vi "Notebooks JSON to LV.vi"(8 "error in (no error)":errorcluster, 11 "Notebooks JSON":string="{\r\n  \"@odata.context\":\"https://www.onenote.com/api/v1.0/$metadata#me/notes/notebooks\",\"value\":[\r\n    {\r\n      \"id\":\"0-C3A40648AD0C9170!191210\",\"self\":\"https://www.onenote.com/api/v1.0/me/notes/notebooks/0-C3A40648AD0C9170!191210\",\"createdTime\":\"2013-11-06T13:59:29.113Z\",\"name\":\"1st Floor Touchscreen\",\"createdBy\":\"Ansom Voodoo\",\"lastModifiedBy\":\"Ansom Voodoo\",\"lastModifiedTime\":\"2018-04-10T18:41:37.72Z\",\"isDefault\":false,\"userRole\":\"Contributor\",\"isShared\":true,\"sectionsUrl\":\"https://www.onenote.com/api/v1.0/me/notes/notebooks/0-C3A40648AD0C9170!191210/sections\",\"sectionGroupsUrl\":\"https://www.onenote.com/api/v1.0/me/notes/notebooks/0-C3A40648AD0C9170!191210/sectionGroups\",\"links\":{\r\n        \"oneNoteClientUrl\":{\r\n          \"href\":\"onenote:https://d.docs.live.net/c3a40648ad0c9170/ansom/Expt.ansom/TouchScreens/1st%20Floor%20Touchscreen\"\r\n        },\"oneNoteWebUrl\":{\r\n          \"href\":\"https://onedrive.live.com/redir.aspx?cid=c3a40648ad0c9170&page=edit&resid=C3A40648AD0C9170!191210&parId=C3A40648AD0C9170!191178\"\r\n        }\r\n      }\r\n    },{\r\n      \"id\":\"0-C3A40648AD0C9170!51956\",\"self\":\"https://www.onenote.com/api/v1.0/me/notes/notebooks/0-C3A40648AD0C9170!51956\",\"createdTime\":\"2013-10-21T12:23:03.47Z\",\"name\":\"2nd Floor TouchScreen\",\"createdBy\":\"Ansom Voodoo\",\"lastModifiedBy\":\"Ansom Voodoo\",\"lastModifiedTime\":\"2018-04-09T20:16:56.763Z\",\"isDefault\":false,\"userRole\":\"Contributor\",\"isShared\":true,\"sectionsUrl\":\"https://www.onenote.com/api/v1.0/me/notes/notebooks/0-C3A40648AD0C9170!51956/sections\",\"sectionGroupsUrl\":\"https://www.onenote.com/api/v1.0/me/notes/notebooks/0-C3A40648AD0C9170!51956/sectionGroups\",\"links\":{\r\n        \"oneNoteClientUrl\":{\r\n          \"href\":\"onenote:https://d.docs.live.net/c3a40648ad0c9170/ansom/Expt.ansom/TouchScreens/2nd%20Floor%20TouchScreen\"\r\n        },\"oneNoteWebUrl\":{\r\n          \"href\":\"https://onedrive.live.com/redir.aspx?cid=c3a40648ad0c9170&page=edit&resid=C3A40648AD0C9170!51956&parId=C3A40648AD0C9170!191178\"\r\n        }\r\n      }\r\n    },{\r\n      \"id\":\"0-C3A40648AD0C9170!196233\",\"self\":\"https://www.onenote.com/api/v1.0/me/notes/notebooks/0-C3A40648AD0C9170!196233\",\"createdTime\":\"2016-01-19T19:51:38.267Z\",\"name\":\"Aaron's Notebook\",\"createdBy\":\"Ansom Voodoo\",\"lastModifiedBy\":\"Ansom Voodoo\",\"lastModifiedTime\":\"2018-04-09T20:16:56.763Z\",\"isDefault\":false,\"userRole\":\"Contributor\",\"isShared\":true,\"sectionsUrl\":\"https://www.onenote.com/api/v1.0/me/notes/notebooks/0-C3A40648AD0C9170!196233/sections\",\"sectionGroupsUrl\":\"https://www.onenote.com/api/v1.0/me/notes/notebooks/0-C3A40648AD0C9170!196233/sectionGroups\",\"links\":{\r\n        \"oneNoteClientUrl\":{\r\n          \"href\":\"onenote:https://d.docs.live.net/c3a40648ad0c9170/ansom/Documents/Aaron's%20Notebook\"\r\n        },\"oneNoteWebUrl\":{\r\n          \"href\":\"https://onedrive.live.com/redir.aspx?cid=c3a40648ad0c9170&page=edit&resid=C3A40648AD0C9170!196233&parId=C3A40648AD0C9170!106\"\r\n        }\r\n      }\r\n    },{\r\n      \"id\":\"0-C3A40648AD0C9170!270355\",\"self\":\"https://www.onenote.com/api/v1.0/me/notes/notebooks/0-C3A40648AD0C9170!270355\",\"createdTime\":\"2017-05-22T17:37:24.137Z\",\"name\":\"Aditi's Lab Notebook\",\"createdBy\":\"Ansom Voodoo\",\"lastModifiedBy\":\"ADITI NETHWEWALA\",\"lastModifiedTime\":\"2018-04-09T21:28:50.163Z\",\"isDefault\":false,\"userRole\":\"Contributor\",\"isShared\":true,\"sectionsUrl\":\"https://www.onenote.com/api/v1.0/me/notes/notebooks/0-C3A40648AD0C9170!270355/sections\",\"sectionGroupsUrl\":\"https://www.onenote.com/api/v1.0/me/notes/notebooks/0-C3A40648AD0C9170!270355/sectionGroups\",\"links\":{\r\n        \"oneNoteClientUrl\":{\r\n          \"href\":\"onenote:https://d.docs.live.net/c3a40648ad0c9170/ansom/Expt.ansom/Personal%20Notebooks/Aditi's%20Lab%20Notebook\"\r\n        },\"oneNoteWebUrl\":{\r\n          \"href\":\"https://onedrive.live.com/redir.aspx?cid=c3a40648ad0c9170&page=edit&resid=C3A40648AD0C9170!270355&parId=C3A40648AD0C9170!131418\"\r\n        }\r\n      }\r\n    },{\r\n      \"id\":\"0-C3A40648AD0C9170!191306\",\"self\":\"https://www.onenote.com/api/v1.0/me/notes/notebooks/0-C3A40648AD0C9170!191306\",\"createdTime\":\"2013-11-12T18:58:51.94Z\",\"name\":\"Agilent\",\"createdBy\":\"Ansom Voodoo\",\"lastModifiedBy\":\"Ansom Voodoo\",\"lastModifiedTime\":\"2018-04-09T20:16:56.763Z\",\"isDefault\":false,\"userRole\":\"Contributor\",\"isShared\":true,\"sectionsUrl\":\"https://www.onenote.com/api/v1.0/me/notes/notebooks/0-C3A40648AD0C9170!191306/sections\",\"sectionGroupsUrl\":\"https://www.onenote.com/api/v1.0/me/notes/notebooks/0-C3A40648AD0C9170!191306/sectionGroups\",\"links\":{\r\n        \"oneNoteClientUrl\":{\r\n          \"href\":\"onenote:https://d.docs.live.net/c3a40648ad0c9170/ansom/Documents/Agilent\"\r\n        },\"oneNoteWebUrl\":{\r\n          \"href\":\"https://onedrive.live.com/redir.aspx?cid=c3a40648ad0c9170&page=edit&resid=C3A40648AD0C9170!191306&parId=C3A40648AD0C9170!106\"\r\n        }\r\n      }\r\n    },{\r\n      \"id\":\"0-C3A40648AD0C9170!20391\",\"self\":\"https://www.onenote.com/api/v1.0/me/notes/notebooks/0-C3A40648AD0C9170!20391\",\"createdTime\":\"2013-10-18T22:42:50.41Z\",\"name\":\"Akash's Lab Notebook\",\"createdBy\":\"Ansom Voodoo\",\"lastModifiedBy\":\"Ansom Voodoo\",\"lastModifiedTime\":\"2015-12-18T17:26:31.19Z\",\"isDefault\":false,\"userRole\":\"Contributor\",\"isShared\":true,\"sectionsUrl\":\"https://www.onenote.com/api/v1.0/me/notes/notebooks/0-C3A40648AD0C9170!20391/sections\",\"sectionGroupsUrl\":\"https://www.onenote.com/api/v1.0/me/notes/notebooks/0-C3A40648AD0C9170!20391/sectionGroups\",\"links\":{\r\n        \"oneNoteClientUrl\":{\r\n          \"href\":\"onenote:https://d.docs.live.net/c3a40648ad0c9170/ansom/Expt.ansom/Personal%20Notebooks/Akash's%20Lab%20Notebook\"\r\n        },\"oneNoteWebUrl\":{\r\n          \"href\":\"https://onedrive.live.com/redir.aspx?cid=c3a40648ad0c9170&page=edit&resid=C3A40648AD0C9170!20391&parId=C3A40648AD0C9170!131418\"\r\n        }\r\n      }\r\n    },{\r\n      \"id\":\"0-C3A40648AD0C9170!191914\",\"self\":\"https://www.onenote.com/api/v1.0/me/notes/notebooks/0-C3A40648AD0C9170!191914\",\"createdTime\":\"2014-05-27T12:41:45.763Z\",\"name\":\"Alexandre's Lab Notebook\",\"createdBy\":\"Ansom Voodoo\",\"lastModifiedBy\":\"Ansom Voodoo\",\"lastModifiedTime\":\"2018-04-09T20:16:56.763Z\",\"isDefault\":false,\"userRole\":\"Contributor\",\"isShared\":true,\"sectionsUrl\":\"https://www.onenote.com/api/v1.0/me/notes/notebooks/0-C3A40648AD0C9170!191914/sections\",\"sectionGroupsUrl\":\"https://www.onenote.com/api/v1.0/me/notes/notebooks/0-C3A40648AD0C9170!191914/sectionGroups\",\"links\":{\r\n        \"oneNoteClientUrl\":{\r\n          \"href\":\"onenote:https://d.docs.live.net/c3a40648ad0c9170/ansom/Expt.ansom/Personal%20Notebooks/Alexandre's%20Lab%20Notebook\"\r\n        },\"oneNoteWebUrl\":{\r\n          \"href\":\"https://onedrive.live.com/redir.aspx?cid=c3a40648ad0c9170&page=edit&resid=C3A40648AD0C9170!191914&parId=C3A40648AD0C9170!131418\"\r\n        }\r\n      }\r\n    },{\r\n      \"id\":\"0-C3A40648AD0C9170!191942\",\"self\":\"https://www.onenote.com/api/v1.0/me/notes/notebooks/0-C3A40648AD0C9170!191942\",\"createdTime\":\"2014-06-06T19:55:15.163Z\",\"name\":\"Anil\",\"createdBy\":\"Ansom Voodoo\",\"lastModifiedBy\":\"Ansom Voodoo\",\"lastModifiedTime\":\"2018-04-09T20:16:56.763Z\",\"isDefault\":false,\"userRole\":\"Contributor\",\"isShared\":true,\"sectionsUrl\":\"https://www.onenote.com/api/v1.0/me/notes/notebooks/0-C3A40648AD0C9170!191942/sections\",\"sectionGroupsUrl\":\"https://www.onenote.com/api/v1.0/me/notes/notebooks/0-C3A40648AD0C9170!191942/sectionGroups\",\"links\":{\r\n        \"oneNoteClientUrl\":{\r\n          \"href\":\"onenote:https://d.docs.live.net/c3a40648ad0c9170/ansom/Expt.ansom/Personal%20Notebooks/Anil\"\r\n        },\"oneNoteWebUrl\":{\r\n          \"href\":\"https://onedrive.live.com/redir.aspx?cid=c3a40648ad0c9170&page=edit&resid=C3A40648AD0C9170!191942&parId=C3A40648AD0C9170!131418\"\r\n        }\r\n      }\r\n    },{\r\n      \"id\":\"0-C3A40648AD0C9170!196663\",\"self\":\"https://www.onenote.com/api/v1.0/me/notes/notebooks/0-C3A40648AD0C9170!196663\",\"createdTime\":\"2016-03-05T02:05:16.6Z\",\"name\":\"Anthony's Lab Notebook\",\"createdBy\":\"Ansom Voodoo\",\"lastModifiedBy\":\"Anthony Tylan-Tyler\",\"lastModifiedTime\":\"2018-04-09T20:16:56.763Z\",\"isDefault\":false,\"userRole\":\"Contributor\",\"isShared\":true,\"sectionsUrl\":\"https://www.onenote.com/api/v1.0/me/notes/notebooks/0-C3A40648AD0C9170!196663/sections\",\"sectionGroupsUrl\":\"https://www.onenote.com/api/v1.0/me/notes/notebooks/0-C3A40648AD0C9170!196663/sectionGroups\",\"links\":{\r\n        \"oneNoteClientUrl\":{\r\n          \"href\":\"onenote:https://d.docs.live.net/c3a40648ad0c9170/ansom/Expt.ansom/Personal%20Notebooks/Anthony's%20Lab%20Notebook\"\r\n        },\"oneNoteWebUrl\":{\r\n          \"href\":\"https://onedrive.live.com/redir.aspx?cid=c3a40648ad0c9170&page=edit&resid=C3A40648AD0C9170!196663&parId=C3A40648AD0C9170!131418\"\r\n        }\r\n      }\r\n    },{\r\n      \"id\":\"0-C3A40648AD0C9170!191247\",\"self\":\"https://www.onenote.com/api/v1.0/me/notes/notebooks/0-C3A40648AD0C9170!191247\",\"createdTime\":\"2013-11-07T19:26:36.61Z\",\"name\":\"Arthur's Lab Notebook\",\"createdBy\":\"Ansom Voodoo\",\"lastModifiedBy\":\"Arthur Li\",\"lastModifiedTime\":\"2018-04-10T22:10:50.757Z\",\"isDefault\":false,\"userRole\":\"Contributor\",\"isShared\":true,\"sectionsUrl\":\"https://www.onenote.com/api/v1.0/me/notes/notebooks/0-C3A40648AD0C9170!191247/sections\",\"sectionGroupsUrl\":\"https://www.onenote.com/api/v1.0/me/notes/notebooks/0-C3A40648AD0C9170!191247/sectionGroups\",\"links\":{\r\n        \"oneNoteClientUrl\":{\r\n          \"href\":\"onenote:https://d.docs.live.net/c3a40648ad0c9170/ansom/Expt.ansom/Personal%20Notebooks/Arthur's%20Lab%20Notebook\"\r\n        },\"oneNoteWebUrl\":{\r\n          \"href\":\"https://onedrive.live.com/redir.aspx?cid=c3a40648ad0c9170&page=edit&resid=C3A40648AD0C9170!191247&parId=C3A40648AD0C9170!131418\"\r\n        }\r\n      }\r\n    },{\r\n      \"id\":\"0-C3A40648AD0C9170!192254\",\"self\":\"https://www.onenote.com/api/v1.0/me/notes/notebooks/0-C3A40648AD0C9170!192254\",\"createdTime\":\"2014-09-09T16:01:39.643Z\",\"name\":\"Au_LAO_STO\",\"createdBy\":\"Ansom Voodoo\",\"lastModifiedBy\":\"Ansom Voodoo\",\"lastModifiedTime\":\"2018-04-09T20:16:56.763Z\",\"isDefault\":false,\"userRole\":\"Contributor\",\"isShared\":true,\"sectionsUrl\":\"https://www.onenote.com/api/v1.0/me/notes/notebooks/0-C3A40648AD0C9170!192254/sections\",\"sectionGroupsUrl\":\"https://www.onenote.com/api/v1.0/me/notes/notebooks/0-C3A40648AD0C9170!192254/sectionGroups\",\"links\":{\r\n        \"oneNoteClientUrl\":{\r\n          \"href\":\"onenote:https://d.docs.live.net/c3a40648ad0c9170/ansom/Expt.ansom/Experiment%20Notebooks/Au_LAO_STO\"\r\n        },\"oneNoteWebUrl\":{\r\n          \"href\":\"https://onedrive.live.com/redir.aspx?cid=c3a40648ad0c9170&page=edit&resid=C3A40648AD0C9170!192254&parId=C3A40648AD0C9170!131421\"\r\n        }\r\n      }\r\n    },{\r\n      \"id\":\"0-C3A40648AD0C9170!191287\",\"self\":\"https://www.onenote.com/api/v1.0/me/notes/notebooks/0-C3A40648AD0C9170!191287\",\"createdTime\":\"2013-11-12T00:23:20.337Z\",\"name\":\"BTO-GaAs-AlGaAs\",\"createdBy\":\"Ansom Voodoo\",\"lastModifiedBy\":\"Giriraj Jnawali\",\"lastModifiedTime\":\"2018-04-09T20:16:56.763Z\",\"isDefault\":false,\"userRole\":\"Contributor\",\"isShared\":true,\"sectionsUrl\":\"https://www.onenote.com/api/v1.0/me/notes/notebooks/0-C3A40648AD0C9170!191287/sections\",\"sectionGroupsUrl\":\"https://www.onenote.com/api/v1.0/me/notes/notebooks/0-C3A40648AD0C9170!191287/sectionGroups\",\"links\":{\r\n        \"oneNoteClientUrl\":{\r\n          \"href\":\"onenote:https://d.docs.live.net/c3a40648ad0c9170/ansom/Expt.ansom/Experiment%20Notebooks/BTO-GaAs-AlGaAs\"\r\n        },\"oneNoteWebUrl\":{\r\n          \"href\":\"https://onedrive.live.com/redir.aspx?cid=c3a40648ad0c9170&page=edit&resid=C3A40648AD0C9170!191287&parId=C3A40648AD0C9170!131421\"\r\n        }\r\n      }\r\n    },{\r\n      \"id\":\"0-C3A40648AD0C9170!272441\",\"self\":\"https://www.onenote.com/api/v1.0/me/notes/notebooks/0-C3A40648AD0C9170!272441\",\"createdTime\":\"2017-09-08T00:22:00.91Z\",\"name\":\"CdO\",\"createdBy\":\"Ansom Voodoo\",\"lastModifiedBy\":\"Ansom Voodoo\",\"lastModifiedTime\":\"2018-04-09T20:16:56.763Z\",\"isDefault\":false,\"userRole\":\"Contributor\",\"isShared\":true,\"sectionsUrl\":\"https://www.onenote.com/api/v1.0/me/notes/notebooks/0-C3A40648AD0C9170!272441/sections\",\"sectionGroupsUrl\":\"https://www.onenote.com/api/v1.0/me/notes/notebooks/0-C3A40648AD0C9170!272441/sectionGroups\",\"links\":{\r\n        \"oneNoteClientUrl\":{\r\n          \"href\":\"onenote:https://d.docs.live.net/c3a40648ad0c9170/ansom/Documents/CdO\"\r\n        },\"oneNoteWebUrl\":{\r\n          \"href\":\"https://onedrive.live.com/redir.aspx?cid=c3a40648ad0c9170&page=edit&resid=C3A40648AD0C9170!272441&parId=C3A40648AD0C9170!106\"\r\n        }\r\n      }\r\n    },{\r\n      \"id\":\"0-962DFAE583894FEA!134\",\"self\":\"https://www.onenote.com/api/v1.0/me/notes/notebooks/0-962DFAE583894FEA!134\",\"createdTime\":\"2017-04-25T19:26:59.437Z\",\"name\":\"Chem Notes 2\",\"createdBy\":\"Joseph Albro\",\"lastModifiedBy\":\"Joseph Albro\",\"lastModifiedTime\":\"2017-11-27T15:09:10.54Z\",\"isDefault\":false,\"userRole\":\"Owner\",\"isShared\":false,\"sectionsUrl\":\"https://www.onenote.com/api/v1.0/me/notes/notebooks/0-962DFAE583894FEA!134/sections\",\"sectionGroupsUrl\":\"https://www.onenote.com/api/v1.0/me/notes/notebooks/0-962DFAE583894FEA!134/sectionGroups\",\"links\":{\r\n        \"oneNoteClientUrl\":{\r\n          \"href\":\"onenote:https://d.docs.live.net/962dfae583894fea/Documents/Chem%20Notes%202\"\r\n        },\"oneNoteWebUrl\":{\r\n          \"href\":\"https://onedrive.live.com/redir.aspx?cid=962dfae583894fea&page=edit&resid=962DFAE583894FEA!134\"\r\n        }\r\n      }\r\n    },{\r\n      \"id\":\"0-C3A40648AD0C9170!191219\",\"self\":\"https://www.onenote.com/api/v1.0/me/notes/notebooks/0-C3A40648AD0C9170!191219\",\"createdTime\":\"2013-11-06T20:13:00.347Z\",\"name\":\"Closed-Cycle 10K (large)\",\"createdBy\":\"Ansom Voodoo\",\"lastModifiedBy\":\"Ansom Voodoo\",\"lastModifiedTime\":\"2018-04-09T20:16:56.763Z\",\"isDefault\":false,\"userRole\":\"Contributor\",\"isShared\":true,\"sectionsUrl\":\"https://www.onenote.com/api/v1.0/me/notes/notebooks/0-C3A40648AD0C9170!191219/sections\",\"sectionGroupsUrl\":\"https://www.onenote.com/api/v1.0/me/notes/notebooks/0-C3A40648AD0C9170!191219/sectionGroups\",\"links\":{\r\n        \"oneNoteClientUrl\":{\r\n          \"href\":\"onenote:https://d.docs.live.net/c3a40648ad0c9170/ansom/Expt.ansom/Instrument%20Notebooks/Closed-Cycle%2010K%20(large)\"\r\n        },\"oneNoteWebUrl\":{\r\n          \"href\":\"https://onedrive.live.com/redir.aspx?cid=c3a40648ad0c9170&page=edit&resid=C3A40648AD0C9170!191219&parId=C3A40648AD0C9170!72393\"\r\n        }\r\n      }\r\n    },{\r\n      \"id\":\"0-C3A40648AD0C9170!191216\",\"self\":\"https://www.onenote.com/api/v1.0/me/notes/notebooks/0-C3A40648AD0C9170!191216\",\"createdTime\":\"2013-11-06T20:05:12.467Z\",\"name\":\"Closed-Cycle 10K (small)\",\"createdBy\":\"Ansom Voodoo\",\"lastModifiedBy\":\"Ansom Voodoo\",\"lastModifiedTime\":\"2018-04-09T20:16:56.763Z\",\"isDefault\":false,\"userRole\":\"Contributor\",\"isShared\":true,\"sectionsUrl\":\"https://www.onenote.com/api/v1.0/me/notes/notebooks/0-C3A40648AD0C9170!191216/sections\",\"sectionGroupsUrl\":\"https://www.onenote.com/api/v1.0/me/notes/notebooks/0-C3A40648AD0C9170!191216/sectionGroups\",\"links\":{\r\n        \"oneNoteClientUrl\":{\r\n          \"href\":\"onenote:https://d.docs.live.net/c3a40648ad0c9170/ansom/Expt.ansom/Instrument%20Notebooks/Closed-Cycle%2010K%20(small)\"\r\n        },\"oneNoteWebUrl\":{\r\n          \"href\":\"https://onedrive.live.com/redir.aspx?cid=c3a40648ad0c9170&page=edit&resid=C3A40648AD0C9170!191216&parId=C3A40648AD0C9170!72393\"\r\n        }\r\n      }\r\n    },{\r\n      \"id\":\"0-C3A40648AD0C9170!191773\",\"self\":\"https://www.onenote.com/api/v1.0/me/notes/notebooks/0-C3A40648AD0C9170!191773\",\"createdTime\":\"2014-04-06T13:26:16.663Z\",\"name\":\"Comments\",\"createdBy\":\"Ansom Voodoo\",\"lastModifiedBy\":\"Dongyue Yang\",\"lastModifiedTime\":\"2018-04-09T20:16:56.763Z\",\"isDefault\":false,\"userRole\":\"Contributor\",\"isShared\":true,\"sectionsUrl\":\"https://www.onenote.com/api/v1.0/me/notes/notebooks/0-C3A40648AD0C9170!191773/sections\",\"sectionGroupsUrl\":\"https://www.onenote.com/api/v1.0/me/notes/notebooks/0-C3A40648AD0C9170!191773/sectionGroups\",\"links\":{\r\n        \"oneNoteClientUrl\":{\r\n          \"href\":\"onenote:https://d.docs.live.net/c3a40648ad0c9170/ansom/Manuscripts.ansom/ZZZ%20Old/GeQD/PRL/Comments\"\r\n        },\"oneNoteWebUrl\":{\r\n          \"href\":\"https://onedrive.live.com/redir.aspx?cid=c3a40648ad0c9170&page=edit&resid=C3A40648AD0C9170!191773&parId=C3A40648AD0C9170!2768\"\r\n        }\r\n      }\r\n    },{\r\n      \"id\":\"0-C3A40648AD0C9170!1114\",\"self\":\"https://www.onenote.com/api/v1.0/me/notes/notebooks/0-C3A40648AD0C9170!1114\",\"createdTime\":\"2013-03-29T18:39:42.773Z\",\"name\":\"Cypher\",\"createdBy\":\"Ansom Voodoo\",\"lastModifiedBy\":\"Ansom Voodoo\",\"lastModifiedTime\":\"2018-04-09T20:16:56.763Z\",\"isDefault\":false,\"userRole\":\"Contributor\",\"isShared\":true,\"sectionsUrl\":\"https://www.onenote.com/api/v1.0/me/notes/notebooks/0-C3A40648AD0C9170!1114/sections\",\"sectionGroupsUrl\":\"https://www.onenote.com/api/v1.0/me/notes/notebooks/0-C3A40648AD0C9170!1114/sectionGroups\",\"links\":{\r\n        \"oneNoteClientUrl\":{\r\n          \"href\":\"onenote:https://d.docs.live.net/c3a40648ad0c9170/ansom/Expt.ansom/Instrument%20Notebooks/Cypher\"\r\n        },\"oneNoteWebUrl\":{\r\n          \"href\":\"https://onedrive.live.com/redir.aspx?cid=c3a40648ad0c9170&page=edit&resid=C3A40648AD0C9170!1114&parId=C3A40648AD0C9170!72393\"\r\n        }\r\n      }\r\n    },{\r\n      \"id\":\"0-C3A40648AD0C9170!191256\",\"self\":\"https://www.onenote.com/api/v1.0/me/notes/notebooks/0-C3A40648AD0C9170!191256\",\"createdTime\":\"2013-11-08T19:33:45.793Z\",\"name\":\"Data Acquisition\",\"createdBy\":\"Ansom Voodoo\",\"lastModifiedBy\":\"Ansom Voodoo\",\"lastModifiedTime\":\"2018-04-09T20:16:56.763Z\",\"isDefault\":false,\"userRole\":\"Contributor\",\"isShared\":true,\"sectionsUrl\":\"https://www.onenote.com/api/v1.0/me/notes/notebooks/0-C3A40648AD0C9170!191256/sections\",\"sectionGroupsUrl\":\"https://www.onenote.com/api/v1.0/me/notes/notebooks/0-C3A40648AD0C9170!191256/sectionGroups\",\"links\":{\r\n        \"oneNoteClientUrl\":{\r\n          \"href\":\"onenote:https://d.docs.live.net/c3a40648ad0c9170/ansom/Expt.ansom/Experiment%20Notebooks/Data%20Acquisition\"\r\n        },\"oneNoteWebUrl\":{\r\n          \"href\":\"https://onedrive.live.com/redir.aspx?cid=c3a40648ad0c9170&page=edit&resid=C3A40648AD0C9170!191256&parId=C3A40648AD0C9170!131421\"\r\n        }\r\n      }\r\n    },{\r\n      \"id\":\"0-C3A40648AD0C9170!191740\",\"self\":\"https://www.onenote.com/api/v1.0/me/notes/notebooks/0-C3A40648AD0C9170!191740\",\"createdTime\":\"2014-03-17T14:39:40.217Z\",\"name\":\"Data reservoir\",\"createdBy\":\"Ansom Voodoo\",\"lastModifiedBy\":\"Ansom Voodoo\",\"lastModifiedTime\":\"2018-04-09T20:16:56.763Z\",\"isDefault\":false,\"userRole\":\"Contributor\",\"isShared\":true,\"sectionsUrl\":\"https://www.onenote.com/api/v1.0/me/notes/notebooks/0-C3A40648AD0C9170!191740/sections\",\"sectionGroupsUrl\":\"https://www.onenote.com/api/v1.0/me/notes/notebooks/0-C3A40648AD0C9170!191740/sectionGroups\",\"links\":{\r\n        \"oneNoteClientUrl\":{\r\n          \"href\":\"onenote:https://d.docs.live.net/c3a40648ad0c9170/ansom/Manuscripts.ansom/ZZZ%20Old/Confined%20wire/Figure/Data%20reservoir\"\r\n        },\"oneNoteWebUrl\":{\r\n          \"href\":\"https://onedrive.live.com/redir.aspx?cid=c3a40648ad0c9170&page=edit&resid=C3A40648AD0C9170!191740&parId=C3A40648AD0C9170!837\"\r\n        }\r\n      }\r\n    },{\r\n      \"id\":\"0-C3A40648AD0C9170!270238\",\"self\":\"https://www.onenote.com/api/v1.0/me/notes/notebooks/0-C3A40648AD0C9170!270238\",\"createdTime\":\"2017-05-17T18:57:08.373Z\",\"name\":\"Dengyu's LabNotebook\",\"createdBy\":\"Ansom Voodoo\",\"lastModifiedBy\":\"Ansom Voodoo\",\"lastModifiedTime\":\"2018-04-10T22:10:39.603Z\",\"isDefault\":false,\"userRole\":\"Contributor\",\"isShared\":true,\"sectionsUrl\":\"https://www.onenote.com/api/v1.0/me/notes/notebooks/0-C3A40648AD0C9170!270238/sections\",\"sectionGroupsUrl\":\"https://www.onenote.com/api/v1.0/me/notes/notebooks/0-C3A40648AD0C9170!270238/sectionGroups\",\"links\":{\r\n        \"oneNoteClientUrl\":{\r\n          \"href\":\"onenote:https://d.docs.live.net/c3a40648ad0c9170/ansom/Documents/Dengyu's%20LabNotebook\"\r\n        },\"oneNoteWebUrl\":{\r\n          \"href\":\"https://onedrive.live.com/redir.aspx?cid=c3a40648ad0c9170&page=edit&resid=C3A40648AD0C9170!270238&parId=C3A40648AD0C9170!106\"\r\n        }\r\n      }\r\n    },{\r\n      \"id\":\"0-C3A40648AD0C9170!198419\",\"self\":\"https://www.onenote.com/api/v1.0/me/notes/notebooks/0-C3A40648AD0C9170!198419\",\"createdTime\":\"2016-06-01T18:30:21.857Z\",\"name\":\"Erin Lab Notebook\",\"createdBy\":\"Ansom Voodoo\",\"lastModifiedBy\":\"Ansom Voodoo\",\"lastModifiedTime\":\"2018-04-09T20:16:56.763Z\",\"isDefault\":false,\"userRole\":\"Contributor\",\"isShared\":true,\"sectionsUrl\":\"https://www.onenote.com/api/v1.0/me/notes/notebooks/0-C3A40648AD0C9170!198419/sections\",\"sectionGroupsUrl\":\"https://www.onenote.com/api/v1.0/me/notes/notebooks/0-C3A40648AD0C9170!198419/sectionGroups\",\"links\":{\r\n        \"oneNoteClientUrl\":{\r\n          \"href\":\"onenote:https://d.docs.live.net/c3a40648ad0c9170/ansom/Expt.ansom/Personal%20Notebooks/Erin%20Lab%20Notebook\"\r\n        },\"oneNoteWebUrl\":{\r\n          \"href\":\"https://onedrive.live.com/redir.aspx?cid=c3a40648ad0c9170&page=edit&resid=C3A40648AD0C9170!198419&parId=C3A40648AD0C9170!131418\"\r\n        }\r\n      }\r\n    },{\r\n      \"id\":\"0-C3A40648AD0C9170!2959\",\"self\":\"https://www.onenote.com/api/v1.0/me/notes/notebooks/0-C3A40648AD0C9170!2959\",\"createdTime\":\"2013-09-22T15:25:50.497Z\",\"name\":\"experiments on grapheneLAOSTO\",\"createdBy\":\"Ansom Voodoo\",\"lastModifiedBy\":\"Ansom Voodoo\",\"lastModifiedTime\":\"2018-04-09T20:16:56.763Z\",\"isDefault\":false,\"userRole\":\"Contributor\",\"isShared\":true,\"sectionsUrl\":\"https://www.onenote.com/api/v1.0/me/notes/notebooks/0-C3A40648AD0C9170!2959/sections\",\"sectionGroupsUrl\":\"https://www.onenote.com/api/v1.0/me/notes/notebooks/0-C3A40648AD0C9170!2959/sectionGroups\",\"links\":{\r\n        \"oneNoteClientUrl\":{\r\n          \"href\":\"onenote:https://d.docs.live.net/c3a40648ad0c9170/ansom/Expt.ansom/Experiment%20Notebooks/experiments%20on%20grapheneLAOSTO\"\r\n        },\"oneNoteWebUrl\":{\r\n          \"href\":\"https://onedrive.live.com/redir.aspx?cid=c3a40648ad0c9170&page=edit&resid=C3A40648AD0C9170!2959&parId=C3A40648AD0C9170!131421\"\r\n        }\r\n      }\r\n    },{\r\n      \"id\":\"0-C3A40648AD0C9170!96055\",\"self\":\"https://www.onenote.com/api/v1.0/me/notes/notebooks/0-C3A40648AD0C9170!96055\",\"createdTime\":\"2013-10-25T17:52:55.833Z\",\"name\":\"Feng_note on MFP3d\",\"createdBy\":\"Ansom Voodoo\",\"lastModifiedBy\":\"Ansom Voodoo\",\"lastModifiedTime\":\"2018-04-09T20:16:56.763Z\",\"isDefault\":false,\"userRole\":\"Contributor\",\"isShared\":true,\"sectionsUrl\":\"https://www.onenote.com/api/v1.0/me/notes/notebooks/0-C3A40648AD0C9170!96055/sections\",\"sectionGroupsUrl\":\"https://www.onenote.com/api/v1.0/me/notes/notebooks/0-C3A40648AD0C9170!96055/sectionGroups\",\"links\":{\r\n        \"oneNoteClientUrl\":{\r\n          \"href\":\"onenote:https://d.docs.live.net/c3a40648ad0c9170/ansom/Documents/Feng_note%20on%20MFP3d\"\r\n        },\"oneNoteWebUrl\":{\r\n          \"href\":\"https://onedrive.live.com/redir.aspx?cid=c3a40648ad0c9170&page=edit&resid=C3A40648AD0C9170!96055&parId=C3A40648AD0C9170!106\"\r\n        }\r\n      }\r\n    },{\r\n      \"id\":\"0-C3A40648AD0C9170!191168\",\"self\":\"https://www.onenote.com/api/v1.0/me/notes/notebooks/0-C3A40648AD0C9170!191168\",\"createdTime\":\"2013-11-05T23:02:21.683Z\",\"name\":\"Feng's Lab Notebook\",\"createdBy\":\"Ansom Voodoo\",\"lastModifiedBy\":\"Ansom Voodoo\",\"lastModifiedTime\":\"2018-04-09T20:16:56.763Z\",\"isDefault\":false,\"userRole\":\"Contributor\",\"isShared\":true,\"sectionsUrl\":\"https://www.onenote.com/api/v1.0/me/notes/notebooks/0-C3A40648AD0C9170!191168/sections\",\"sectionGroupsUrl\":\"https://www.onenote.com/api/v1.0/me/notes/notebooks/0-C3A40648AD0C9170!191168/sectionGroups\",\"links\":{\r\n        \"oneNoteClientUrl\":{\r\n          \"href\":\"onenote:https://d.docs.live.net/c3a40648ad0c9170/ansom/Expt.ansom/Personal%20Notebooks/Feng's%20Lab%20Notebook\"\r\n        },\"oneNoteWebUrl\":{\r\n          \"href\":\"https://onedrive.live.com/redir.aspx?cid=c3a40648ad0c9170&page=edit&resid=C3A40648AD0C9170!191168&parId=C3A40648AD0C9170!131418\"\r\n        }\r\n      }\r\n    },{\r\n      \"id\":\"0-C3A40648AD0C9170!191172\",\"self\":\"https://www.onenote.com/api/v1.0/me/notes/notebooks/0-C3A40648AD0C9170!191172\",\"createdTime\":\"2013-11-06T13:12:16.157Z\",\"name\":\"First Floor Touch\",\"createdBy\":\"Ansom Voodoo\",\"lastModifiedBy\":\"Ansom Voodoo\",\"lastModifiedTime\":\"2018-04-09T20:16:56.763Z\",\"isDefault\":false,\"userRole\":\"Contributor\",\"isShared\":true,\"sectionsUrl\":\"https://www.onenote.com/api/v1.0/me/notes/notebooks/0-C3A40648AD0C9170!191172/sections\",\"sectionGroupsUrl\":\"https://www.onenote.com/api/v1.0/me/notes/notebooks/0-C3A40648AD0C9170!191172/sectionGroups\",\"links\":{\r\n        \"oneNoteClientUrl\":{\r\n          \"href\":\"onenote:https://d.docs.live.net/c3a40648ad0c9170/ansom/Documents/First%20Floor%20Touch\"\r\n        },\"oneNoteWebUrl\":{\r\n          \"href\":\"https://onedrive.live.com/redir.aspx?cid=c3a40648ad0c9170&page=edit&resid=C3A40648AD0C9170!191172&parId=C3A40648AD0C9170!106\"\r\n        }\r\n      }\r\n    },{\r\n      \"id\":\"0-C3A40648AD0C9170!196438\",\"self\":\"https://www.onenote.com/api/v1.0/me/notes/notebooks/0-C3A40648AD0C9170!196438\",\"createdTime\":\"2016-01-29T20:18:55.9Z\",\"name\":\"Garrison Notebook\",\"createdBy\":\"Ansom Voodoo\",\"lastModifiedBy\":\"Ansom Voodoo\",\"lastModifiedTime\":\"2018-04-09T20:16:56.763Z\",\"isDefault\":false,\"userRole\":\"Contributor\",\"isShared\":true,\"sectionsUrl\":\"https://www.onenote.com/api/v1.0/me/notes/notebooks/0-C3A40648AD0C9170!196438/sections\",\"sectionGroupsUrl\":\"https://www.onenote.com/api/v1.0/me/notes/notebooks/0-C3A40648AD0C9170!196438/sectionGroups\",\"links\":{\r\n        \"oneNoteClientUrl\":{\r\n          \"href\":\"onenote:https://d.docs.live.net/c3a40648ad0c9170/ansom/Documents/Garrison%20Notebook\"\r\n        },\"oneNoteWebUrl\":{\r\n          \"href\":\"https://onedrive.live.com/redir.aspx?cid=c3a40648ad0c9170&page=edit&resid=C3A40648AD0C9170!196438&parId=C3A40648AD0C9170!106\"\r\n        }\r\n      }\r\n    },{\r\n      \"id\":\"0-C3A40648AD0C9170!269616\",\"self\":\"https://www.onenote.com/api/v1.0/me/notes/notebooks/0-C3A40648AD0C9170!269616\",\"createdTime\":\"2017-04-04T21:30:19.743Z\",\"name\":\"GCO_Project\",\"createdBy\":\"Ansom Voodoo\",\"lastModifiedBy\":\"Ansom Voodoo\",\"lastModifiedTime\":\"2018-04-10T22:43:35.643Z\",\"isDefault\":false,\"userRole\":\"Contributor\",\"isShared\":true,\"sectionsUrl\":\"https://www.onenote.com/api/v1.0/me/notes/notebooks/0-C3A40648AD0C9170!269616/sections\",\"sectionGroupsUrl\":\"https://www.onenote.com/api/v1.0/me/notes/notebooks/0-C3A40648AD0C9170!269616/sectionGroups\",\"links\":{\r\n        \"oneNoteClientUrl\":{\r\n          \"href\":\"onenote:https://d.docs.live.net/c3a40648ad0c9170/ansom/Documents/GCO_Project\"\r\n        },\"oneNoteWebUrl\":{\r\n          \"href\":\"https://onedrive.live.com/redir.aspx?cid=c3a40648ad0c9170&page=edit&resid=C3A40648AD0C9170!269616&parId=C3A40648AD0C9170!106\"\r\n        }\r\n      }\r\n    },{\r\n      \"id\":\"0-C3A40648AD0C9170!208841\",\"self\":\"https://www.onenote.com/api/v1.0/me/notes/notebooks/0-C3A40648AD0C9170!208841\",\"createdTime\":\"2016-07-01T20:09:49.177Z\",\"name\":\"Graphene growth\",\"createdBy\":\"Ansom Voodoo\",\"lastModifiedBy\":\"Arthur Li\",\"lastModifiedTime\":\"2018-04-09T20:16:56.763Z\",\"isDefault\":false,\"userRole\":\"Contributor\",\"isShared\":true,\"sectionsUrl\":\"https://www.onenote.com/api/v1.0/me/notes/notebooks/0-C3A40648AD0C9170!208841/sections\",\"sectionGroupsUrl\":\"https://www.onenote.com/api/v1.0/me/notes/notebooks/0-C3A40648AD0C9170!208841/sectionGroups\",\"links\":{\r\n        \"oneNoteClientUrl\":{\r\n          \"href\":\"onenote:https://d.docs.live.net/c3a40648ad0c9170/ansom/Expt.ansom/Personal%20Notebooks/Graphene%20growth\"\r\n        },\"oneNoteWebUrl\":{\r\n          \"href\":\"https://onedrive.live.com/redir.aspx?cid=c3a40648ad0c9170&page=edit&resid=C3A40648AD0C9170!208841&parId=C3A40648AD0C9170!131418\"\r\n        }\r\n      }\r\n    },{\r\n      \"id\":\"0-C3A40648AD0C9170!2963\",\"self\":\"https://www.onenote.com/api/v1.0/me/notes/notebooks/0-C3A40648AD0C9170!2963\",\"createdTime\":\"2013-09-22T15:32:06.73Z\",\"name\":\"Graphene.LAO.STO\",\"createdBy\":\"Ansom Voodoo\",\"lastModifiedBy\":\"Arthur Li\",\"lastModifiedTime\":\"2018-04-09T20:16:56.763Z\",\"isDefault\":false,\"userRole\":\"Contributor\",\"isShared\":true,\"sectionsUrl\":\"https://www.onenote.com/api/v1.0/me/notes/notebooks/0-C3A40648AD0C9170!2963/sections\",\"sectionGroupsUrl\":\"https://www.onenote.com/api/v1.0/me/notes/notebooks/0-C3A40648AD0C9170!2963/sectionGroups\",\"links\":{\r\n        \"oneNoteClientUrl\":{\r\n          \"href\":\"onenote:https://d.docs.live.net/c3a40648ad0c9170/ansom/Expt.ansom/Experiment%20Notebooks/Graphene.LAO.STO\"\r\n        },\"oneNoteWebUrl\":{\r\n          \"href\":\"https://onedrive.live.com/redir.aspx?cid=c3a40648ad0c9170&page=edit&resid=C3A40648AD0C9170!2963&parId=C3A40648AD0C9170!131421\"\r\n        }\r\n      }\r\n    },{\r\n      \"id\":\"0-C3A40648AD0C9170!192197\",\"self\":\"https://www.onenote.com/api/v1.0/me/notes/notebooks/0-C3A40648AD0C9170!192197\",\"createdTime\":\"2014-08-20T15:11:01.43Z\",\"name\":\"graphene.LAO.STO growth.characterization\",\"createdBy\":\"Ansom Voodoo\",\"lastModifiedBy\":\"Ansom Voodoo\",\"lastModifiedTime\":\"2018-04-09T20:16:56.763Z\",\"isDefault\":false,\"userRole\":\"Contributor\",\"isShared\":true,\"sectionsUrl\":\"https://www.onenote.com/api/v1.0/me/notes/notebooks/0-C3A40648AD0C9170!192197/sections\",\"sectionGroupsUrl\":\"https://www.onenote.com/api/v1.0/me/notes/notebooks/0-C3A40648AD0C9170!192197/sectionGroups\",\"links\":{\r\n        \"oneNoteClientUrl\":{\r\n          \"href\":\"onenote:https://d.docs.live.net/c3a40648ad0c9170/ansom/Expt.ansom/Experiment%20Notebooks/graphene.LAO.STO%20growth.characterization\"\r\n        },\"oneNoteWebUrl\":{\r\n          \"href\":\"https://onedrive.live.com/redir.aspx?cid=c3a40648ad0c9170&page=edit&resid=C3A40648AD0C9170!192197&parId=C3A40648AD0C9170!131421\"\r\n        }\r\n      }\r\n    },{\r\n      \"id\":\"0-C3A40648AD0C9170!191952\",\"self\":\"https://www.onenote.com/api/v1.0/me/notes/notebooks/0-C3A40648AD0C9170!191952\",\"createdTime\":\"2014-06-09T21:42:15.157Z\",\"name\":\"Ishan Levy Labboook\",\"createdBy\":\"Ansom Voodoo\",\"lastModifiedBy\":\"Ansom Voodoo\",\"lastModifiedTime\":\"2018-04-09T20:16:56.763Z\",\"isDefault\":false,\"userRole\":\"Contributor\",\"isShared\":true,\"sectionsUrl\":\"https://www.onenote.com/api/v1.0/me/notes/notebooks/0-C3A40648AD0C9170!191952/sections\",\"sectionGroupsUrl\":\"https://www.onenote.com/api/v1.0/me/notes/notebooks/0-C3A40648AD0C9170!191952/sectionGroups\",\"links\":{\r\n        \"oneNoteClientUrl\":{\r\n          \"href\":\"onenote:https://d.docs.live.net/c3a40648ad0c9170/ansom/Documents/Ishan%20Levy%20Labboook\"\r\n        },\"oneNoteWebUrl\":{\r\n          \"href\":\"https://onedrive.live.com/redir.aspx?cid=c3a40648ad0c9170&page=edit&resid=C3A40648AD0C9170!191952&parId=C3A40648AD0C9170!106\"\r\n        }\r\n      }\r\n    },{\r\n      \"id\":\"0-C3A40648AD0C9170!191387\",\"self\":\"https://www.onenote.com/api/v1.0/me/notes/notebooks/0-C3A40648AD0C9170!191387\",\"createdTime\":\"2013-12-04T18:59:10.48Z\",\"name\":\"JEOL\",\"createdBy\":\"Ansom Voodoo\",\"lastModifiedBy\":\"Ansom Voodoo\",\"lastModifiedTime\":\"2018-04-09T20:16:56.763Z\",\"isDefault\":false,\"userRole\":\"Contributor\",\"isShared\":true,\"sectionsUrl\":\"https://www.onenote.com/api/v1.0/me/notes/notebooks/0-C3A40648AD0C9170!191387/sections\",\"sectionGroupsUrl\":\"https://www.onenote.com/api/v1.0/me/notes/notebooks/0-C3A40648AD0C9170!191387/sectionGroups\",\"links\":{\r\n        \"oneNoteClientUrl\":{\r\n          \"href\":\"onenote:https://d.docs.live.net/c3a40648ad0c9170/ansom/Expt.ansom/Instrument%20Notebooks/JEOL\"\r\n        },\"oneNoteWebUrl\":{\r\n          \"href\":\"https://onedrive.live.com/redir.aspx?cid=c3a40648ad0c9170&page=edit&resid=C3A40648AD0C9170!191387&parId=C3A40648AD0C9170!72393\"\r\n        }\r\n      }\r\n    },{\r\n      \"id\":\"0-C3A40648AD0C9170!194543\",\"self\":\"https://www.onenote.com/api/v1.0/me/notes/notebooks/0-C3A40648AD0C9170!194543\",\"createdTime\":\"2015-07-05T17:41:31.9Z\",\"name\":\"jeremy.levy Notebook\",\"createdBy\":\"Ansom Voodoo\",\"lastModifiedBy\":\"Jeremy Levy\",\"lastModifiedTime\":\"2018-04-09T20:16:56.763Z\",\"isDefault\":false,\"userRole\":\"Contributor\",\"isShared\":true,\"sectionsUrl\":\"https://www.onenote.com/api/v1.0/me/notes/notebooks/0-C3A40648AD0C9170!194543/sections\",\"sectionGroupsUrl\":\"https://www.onenote.com/api/v1.0/me/notes/notebooks/0-C3A40648AD0C9170!194543/sectionGroups\",\"links\":{\r\n        \"oneNoteClientUrl\":{\r\n          \"href\":\"onenote:https://d.docs.live.net/c3a40648ad0c9170/ansom/Expt.ansom/Personal%20Notebooks/jeremy.levy%20Notebook\"\r\n        },\"oneNoteWebUrl\":{\r\n          \"href\":\"https://onedrive.live.com/redir.aspx?cid=c3a40648ad0c9170&page=edit&resid=C3A40648AD0C9170!194543&parId=C3A40648AD0C9170!131418\"\r\n        }\r\n      }\r\n    },{\r\n      \"id\":\"0-C3A40648AD0C9170!193671\",\"self\":\"https://www.onenote.com/api/v1.0/me/notes/notebooks/0-C3A40648AD0C9170!193671\",\"createdTime\":\"2015-01-23T21:21:54.723Z\",\"name\":\"Jessica's Lab Notebook\",\"createdBy\":\"Ansom Voodoo\",\"lastModifiedBy\":\"Ansom Voodoo\",\"lastModifiedTime\":\"2018-04-10T17:57:06.043Z\",\"isDefault\":false,\"userRole\":\"Contributor\",\"isShared\":true,\"sectionsUrl\":\"https://www.onenote.com/api/v1.0/me/notes/notebooks/0-C3A40648AD0C9170!193671/sections\",\"sectionGroupsUrl\":\"https://www.onenote.com/api/v1.0/me/notes/notebooks/0-C3A40648AD0C9170!193671/sectionGroups\",\"links\":{\r\n        \"oneNoteClientUrl\":{\r\n          \"href\":\"onenote:https://d.docs.live.net/c3a40648ad0c9170/ansom/Expt.ansom/Personal%20Notebooks/Jessica's%20Lab%20Notebook\"\r\n        },\"oneNoteWebUrl\":{\r\n          \"href\":\"https://onedrive.live.com/redir.aspx?cid=c3a40648ad0c9170&page=edit&resid=C3A40648AD0C9170!193671&parId=C3A40648AD0C9170!131418\"\r\n        }\r\n      }\r\n    },{\r\n      \"id\":\"0-C3A40648AD0C9170!208803\",\"self\":\"https://www.onenote.com/api/v1.0/me/notes/notebooks/0-C3A40648AD0C9170!208803\",\"createdTime\":\"2016-06-30T17:30:17.65Z\",\"name\":\"Jim Mangum\",\"createdBy\":\"Ansom Voodoo\",\"lastModifiedBy\":\"\",\"lastModifiedTime\":\"2018-04-09T20:16:56.763Z\",\"isDefault\":false,\"userRole\":\"Contributor\",\"isShared\":true,\"sectionsUrl\":\"https://www.onenote.com/api/v1.0/me/notes/notebooks/0-C3A40648AD0C9170!208803/sections\",\"sectionGroupsUrl\":\"https://www.onenote.com/api/v1.0/me/notes/notebooks/0-C3A40648AD0C9170!208803/sectionGroups\",\"links\":{\r\n        \"oneNoteClientUrl\":{\r\n          \"href\":\"onenote:https://d.docs.live.net/c3a40648ad0c9170/ansom/Expt.ansom/Personal%20Notebooks/Jim%20Mangum\"\r\n        },\"oneNoteWebUrl\":{\r\n          \"href\":\"https://onedrive.live.com/redir.aspx?cid=c3a40648ad0c9170&page=edit&resid=C3A40648AD0C9170!208803&parId=C3A40648AD0C9170!131418\"\r\n        }\r\n      }\r\n    },{\r\n      \"id\":\"0-962DFAE583894FEA!170\",\"self\":\"https://www.onenote.com/api/v1.0/me/notes/notebooks/0-962DFAE583894FEA!170\",\"createdTime\":\"2017-06-18T21:32:44.213Z\",\"name\":\"Joe Albro\",\"createdBy\":\"Joseph Albro\",\"lastModifiedBy\":\"Joseph Albro\",\"lastModifiedTime\":\"2018-03-16T23:09:34.713Z\",\"isDefault\":false,\"userRole\":\"Owner\",\"isShared\":false,\"sectionsUrl\":\"https://www.onenote.com/api/v1.0/me/notes/notebooks/0-962DFAE583894FEA!170/sections\",\"sectionGroupsUrl\":\"https://www.onenote.com/api/v1.0/me/notes/notebooks/0-962DFAE583894FEA!170/sectionGroups\",\"links\":{\r\n        \"oneNoteClientUrl\":{\r\n          \"href\":\"onenote:https://d.docs.live.net/962dfae583894fea/Documents/Joe%20Albro\"\r\n        },\"oneNoteWebUrl\":{\r\n          \"href\":\"https://onedrive.live.com/redir.aspx?cid=962dfae583894fea&page=edit&resid=962DFAE583894FEA!170\"\r\n        }\r\n      }\r\n    },{\r\n      \"id\":\"0-962DFAE583894FEA!116\",\"self\":\"https://www.onenote.com/api/v1.0/me/notes/notebooks/0-962DFAE583894FEA!116\",\"createdTime\":\"2017-04-23T19:40:16.197Z\",\"name\":\"Joe Albro (1)\",\"createdBy\":\"Joseph Albro\",\"lastModifiedBy\":\"Joseph Albro\",\"lastModifiedTime\":\"2017-11-27T15:09:03.303Z\",\"isDefault\":false,\"userRole\":\"Owner\",\"isShared\":false,\"sectionsUrl\":\"https://www.onenote.com/api/v1.0/me/notes/notebooks/0-962DFAE583894FEA!116/sections\",\"sectionGroupsUrl\":\"https://www.onenote.com/api/v1.0/me/notes/notebooks/0-962DFAE583894FEA!116/sectionGroups\",\"links\":{\r\n        \"oneNoteClientUrl\":{\r\n          \"href\":\"onenote:https://d.docs.live.net/962dfae583894fea/Documents/Joe%20Albro%20(1)\"\r\n        },\"oneNoteWebUrl\":{\r\n          \"href\":\"https://onedrive.live.com/redir.aspx?cid=962dfae583894fea&page=edit&resid=962DFAE583894FEA!116\"\r\n        }\r\n      }\r\n    },{\r\n      \"id\":\"0-C3A40648AD0C9170!184715\",\"self\":\"https://www.onenote.com/api/v1.0/me/notes/notebooks/0-C3A40648AD0C9170!184715\",\"createdTime\":\"2013-11-04T20:31:19.34Z\",\"name\":\"Joe's Lab Notebook\",\"createdBy\":\"Ansom Voodoo\",\"lastModifiedBy\":\"Yuhe Tang\",\"lastModifiedTime\":\"2018-04-09T20:16:56.763Z\",\"isDefault\":false,\"userRole\":\"Contributor\",\"isShared\":true,\"sectionsUrl\":\"https://www.onenote.com/api/v1.0/me/notes/notebooks/0-C3A40648AD0C9170!184715/sections\",\"sectionGroupsUrl\":\"https://www.onenote.com/api/v1.0/me/notes/notebooks/0-C3A40648AD0C9170!184715/sectionGroups\",\"links\":{\r\n        \"oneNoteClientUrl\":{\r\n          \"href\":\"onenote:https://d.docs.live.net/c3a40648ad0c9170/ansom/Expt.ansom/Personal%20Notebooks/Alumni/Joe's%20Lab%20Notebook\"\r\n        },\"oneNoteWebUrl\":{\r\n          \"href\":\"https://onedrive.live.com/redir.aspx?cid=c3a40648ad0c9170&page=edit&resid=C3A40648AD0C9170!184715&parId=C3A40648AD0C9170!194471\"\r\n        }\r\n      }\r\n    },{\r\n      \"id\":\"0-C3A40648AD0C9170!193945\",\"self\":\"https://www.onenote.com/api/v1.0/me/notes/notebooks/0-C3A40648AD0C9170!193945\",\"createdTime\":\"2015-03-19T20:55:49.147Z\",\"name\":\"LAO_MBE grown STO\",\"createdBy\":\"Ansom Voodoo\",\"lastModifiedBy\":\"mengchen huang\",\"lastModifiedTime\":\"2018-04-09T20:16:56.763Z\",\"isDefault\":false,\"userRole\":\"Contributor\",\"isShared\":true,\"sectionsUrl\":\"https://www.onenote.com/api/v1.0/me/notes/notebooks/0-C3A40648AD0C9170!193945/sections\",\"sectionGroupsUrl\":\"https://www.onenote.com/api/v1.0/me/notes/notebooks/0-C3A40648AD0C9170!193945/sectionGroups\",\"links\":{\r\n        \"oneNoteClientUrl\":{\r\n          \"href\":\"onenote:https://d.docs.live.net/c3a40648ad0c9170/ansom/Expt.ansom/Experiment%20Notebooks/LAO_MBE%20grown%20STO\"\r\n        },\"oneNoteWebUrl\":{\r\n          \"href\":\"https://onedrive.live.com/redir.aspx?cid=c3a40648ad0c9170&page=edit&resid=C3A40648AD0C9170!193945&parId=C3A40648AD0C9170!131421\"\r\n        }\r\n      }\r\n    },{\r\n      \"id\":\"0-C3A40648AD0C9170!272997\",\"self\":\"https://www.onenote.com/api/v1.0/me/notes/notebooks/0-C3A40648AD0C9170!272997\",\"createdTime\":\"2017-11-10T22:05:48.193Z\",\"name\":\"Leena's Notebook\",\"createdBy\":\"Ansom Voodoo\",\"lastModifiedBy\":\"Ansom Voodoo\",\"lastModifiedTime\":\"2018-04-10T00:44:08.18Z\",\"isDefault\":false,\"userRole\":\"Contributor\",\"isShared\":true,\"sectionsUrl\":\"https://www.onenote.com/api/v1.0/me/notes/notebooks/0-C3A40648AD0C9170!272997/sections\",\"sectionGroupsUrl\":\"https://www.onenote.com/api/v1.0/me/notes/notebooks/0-C3A40648AD0C9170!272997/sectionGroups\",\"links\":{\r\n        \"oneNoteClientUrl\":{\r\n          \"href\":\"onenote:https://d.docs.live.net/c3a40648ad0c9170/ansom/Expt.ansom/Personal%20Notebooks/Leena's%20Notebook\"\r\n        },\"oneNoteWebUrl\":{\r\n          \"href\":\"https://onedrive.live.com/redir.aspx?cid=c3a40648ad0c9170&page=edit&resid=C3A40648AD0C9170!272997&parId=C3A40648AD0C9170!131418\"\r\n        }\r\n      }\r\n    },{\r\n      \"id\":\"0-C3A40648AD0C9170!191020\",\"self\":\"https://www.onenote.com/api/v1.0/me/notes/notebooks/0-C3A40648AD0C9170!191020\",\"createdTime\":\"2013-11-05T19:44:43.453Z\",\"name\":\"Leiden 18 T\",\"createdBy\":\"Ansom Voodoo\",\"lastModifiedBy\":\"Megan Kirkendall\",\"lastModifiedTime\":\"2018-04-10T12:21:58.307Z\",\"isDefault\":false,\"userRole\":\"Contributor\",\"isShared\":true,\"sectionsUrl\":\"https://www.onenote.com/api/v1.0/me/notes/notebooks/0-C3A40648AD0C9170!191020/sections\",\"sectionGroupsUrl\":\"https://www.onenote.com/api/v1.0/me/notes/notebooks/0-C3A40648AD0C9170!191020/sectionGroups\",\"links\":{\r\n        \"oneNoteClientUrl\":{\r\n          \"href\":\"onenote:https://d.docs.live.net/c3a40648ad0c9170/ansom/Expt.ansom/Instrument%20Notebooks/Leiden%20mnk/Leiden%2018%20T\"\r\n        },\"oneNoteWebUrl\":{\r\n          \"href\":\"https://onedrive.live.com/redir.aspx?cid=c3a40648ad0c9170&page=edit&resid=C3A40648AD0C9170!191020&parId=C3A40648AD0C9170!195036\"\r\n        }\r\n      }\r\n    },{\r\n      \"id\":\"0-C3A40648AD0C9170!166661\",\"self\":\"https://www.onenote.com/api/v1.0/me/notes/notebooks/0-C3A40648AD0C9170!166661\",\"createdTime\":\"2013-11-02T13:13:07.413Z\",\"name\":\"Leiden CF\",\"createdBy\":\"Ansom Voodoo\",\"lastModifiedBy\":\"Megan Kirkendall\",\"lastModifiedTime\":\"2018-04-10T22:42:23.08Z\",\"isDefault\":false,\"userRole\":\"Contributor\",\"isShared\":true,\"sectionsUrl\":\"https://www.onenote.com/api/v1.0/me/notes/notebooks/0-C3A40648AD0C9170!166661/sections\",\"sectionGroupsUrl\":\"https://www.onenote.com/api/v1.0/me/notes/notebooks/0-C3A40648AD0C9170!166661/sectionGroups\",\"links\":{\r\n        \"oneNoteClientUrl\":{\r\n          \"href\":\"onenote:https://d.docs.live.net/c3a40648ad0c9170/ansom/Expt.ansom/Instrument%20Notebooks/Leiden%20CF\"\r\n        },\"oneNoteWebUrl\":{\r\n          \"href\":\"https://onedrive.live.com/redir.aspx?cid=c3a40648ad0c9170&page=edit&resid=C3A40648AD0C9170!166661&parId=C3A40648AD0C9170!72393\"\r\n        }\r\n      }\r\n    },{\r\n      \"id\":\"0-C3A40648AD0C9170!191722\",\"self\":\"https://www.onenote.com/api/v1.0/me/notes/notebooks/0-C3A40648AD0C9170!191722\",\"createdTime\":\"2014-03-12T18:28:06.84Z\",\"name\":\"Levy - Frolov Low T Instrumentation\",\"createdBy\":\"Ansom Voodoo\",\"lastModifiedBy\":\"Ansom Voodoo\",\"lastModifiedTime\":\"2018-04-09T20:16:56.763Z\",\"isDefault\":false,\"userRole\":\"Contributor\",\"isShared\":true,\"sectionsUrl\":\"https://www.onenote.com/api/v1.0/me/notes/notebooks/0-C3A40648AD0C9170!191722/sections\",\"sectionGroupsUrl\":\"https://www.onenote.com/api/v1.0/me/notes/notebooks/0-C3A40648AD0C9170!191722/sectionGroups\",\"links\":{\r\n        \"oneNoteClientUrl\":{\r\n          \"href\":\"onenote:https://d.docs.live.net/c3a40648ad0c9170/ansom/Expt.ansom/Instrument%20Notebooks/Levy%20-%20Frolov%20Low%20T%20Instrumentation\"\r\n        },\"oneNoteWebUrl\":{\r\n          \"href\":\"https://onedrive.live.com/redir.aspx?cid=c3a40648ad0c9170&page=edit&resid=C3A40648AD0C9170!191722&parId=C3A40648AD0C9170!72393\"\r\n        }\r\n      }\r\n    },{\r\n      \"id\":\"0-C3A40648AD0C9170!160788\",\"self\":\"https://www.onenote.com/api/v1.0/me/notes/notebooks/0-C3A40648AD0C9170!160788\",\"createdTime\":\"2013-11-01T19:48:12.533Z\",\"name\":\"Lucy's Lab Notebook\",\"createdBy\":\"Ansom Voodoo\",\"lastModifiedBy\":\"Lu Chen\",\"lastModifiedTime\":\"2018-04-09T20:16:56.763Z\",\"isDefault\":false,\"userRole\":\"Contributor\",\"isShared\":true,\"sectionsUrl\":\"https://www.onenote.com/api/v1.0/me/notes/notebooks/0-C3A40648AD0C9170!160788/sections\",\"sectionGroupsUrl\":\"https://www.onenote.com/api/v1.0/me/notes/notebooks/0-C3A40648AD0C9170!160788/sectionGroups\",\"links\":{\r\n        \"oneNoteClientUrl\":{\r\n          \"href\":\"onenote:https://d.docs.live.net/c3a40648ad0c9170/ansom/Expt.ansom/Personal%20Notebooks/Lucy's%20Lab%20Notebook\"\r\n        },\"oneNoteWebUrl\":{\r\n          \"href\":\"https://onedrive.live.com/redir.aspx?cid=c3a40648ad0c9170&page=edit&resid=C3A40648AD0C9170!160788&parId=C3A40648AD0C9170!131418\"\r\n        }\r\n      }\r\n    },{\r\n      \"id\":\"0-C3A40648AD0C9170!132401\",\"self\":\"https://www.onenote.com/api/v1.0/me/notes/notebooks/0-C3A40648AD0C9170!132401\",\"createdTime\":\"2013-10-29T19:56:19.613Z\",\"name\":\"Megan's Lab Notebook\",\"createdBy\":\"Ansom Voodoo\",\"lastModifiedBy\":\"Megan Kirkendall\",\"lastModifiedTime\":\"2018-04-10T16:57:53.4Z\",\"isDefault\":false,\"userRole\":\"Contributor\",\"isShared\":true,\"sectionsUrl\":\"https://www.onenote.com/api/v1.0/me/notes/notebooks/0-C3A40648AD0C9170!132401/sections\",\"sectionGroupsUrl\":\"https://www.onenote.com/api/v1.0/me/notes/notebooks/0-C3A40648AD0C9170!132401/sectionGroups\",\"links\":{\r\n        \"oneNoteClientUrl\":{\r\n          \"href\":\"onenote:https://d.docs.live.net/c3a40648ad0c9170/ansom/Expt.ansom/Personal%20Notebooks/Megan's%20Lab%20Notebook\"\r\n        },\"oneNoteWebUrl\":{\r\n          \"href\":\"https://onedrive.live.com/redir.aspx?cid=c3a40648ad0c9170&page=edit&resid=C3A40648AD0C9170!132401&parId=C3A40648AD0C9170!131418\"\r\n        }\r\n      }\r\n    },{\r\n      \"id\":\"0-C3A40648AD0C9170!191946\",\"self\":\"https://www.onenote.com/api/v1.0/me/notes/notebooks/0-C3A40648AD0C9170!191946\",\"createdTime\":\"2014-06-06T23:10:31.72Z\",\"name\":\"MFP3D\",\"createdBy\":\"Ansom Voodoo\",\"lastModifiedBy\":\"Ansom Voodoo\",\"lastModifiedTime\":\"2018-04-09T20:16:56.763Z\",\"isDefault\":false,\"userRole\":\"Contributor\",\"isShared\":true,\"sectionsUrl\":\"https://www.onenote.com/api/v1.0/me/notes/notebooks/0-C3A40648AD0C9170!191946/sections\",\"sectionGroupsUrl\":\"https://www.onenote.com/api/v1.0/me/notes/notebooks/0-C3A40648AD0C9170!191946/sectionGroups\",\"links\":{\r\n        \"oneNoteClientUrl\":{\r\n          \"href\":\"onenote:https://d.docs.live.net/c3a40648ad0c9170/ansom/Expt.ansom/Instrument%20Notebooks/MFP3D\"\r\n        },\"oneNoteWebUrl\":{\r\n          \"href\":\"https://onedrive.live.com/redir.aspx?cid=c3a40648ad0c9170&page=edit&resid=C3A40648AD0C9170!191946&parId=C3A40648AD0C9170!72393\"\r\n        }\r\n      }\r\n    },{\r\n      \"id\":\"0-C3A40648AD0C9170!192115\",\"self\":\"https://www.onenote.com/api/v1.0/me/notes/notebooks/0-C3A40648AD0C9170!192115\",\"createdTime\":\"2014-07-24T19:29:28.203Z\",\"name\":\"Michael's Lab Notebook\",\"createdBy\":\"Ansom Voodoo\",\"lastModifiedBy\":\"Yuhe Tang\",\"lastModifiedTime\":\"2018-04-09T20:16:56.763Z\",\"isDefault\":false,\"userRole\":\"Contributor\",\"isShared\":true,\"sectionsUrl\":\"https://www.onenote.com/api/v1.0/me/notes/notebooks/0-C3A40648AD0C9170!192115/sections\",\"sectionGroupsUrl\":\"https://www.onenote.com/api/v1.0/me/notes/notebooks/0-C3A40648AD0C9170!192115/sectionGroups\",\"links\":{\r\n        \"oneNoteClientUrl\":{\r\n          \"href\":\"onenote:https://d.docs.live.net/c3a40648ad0c9170/ansom/Expt.ansom/Personal%20Notebooks/Alumni/Michael's%20Lab%20Notebook\"\r\n        },\"oneNoteWebUrl\":{\r\n          \"href\":\"https://onedrive.live.com/redir.aspx?cid=c3a40648ad0c9170&page=edit&resid=C3A40648AD0C9170!192115&parId=C3A40648AD0C9170!194471\"\r\n        }\r\n      }\r\n    },{\r\n      \"id\":\"0-C3A40648AD0C9170!194485\",\"self\":\"https://www.onenote.com/api/v1.0/me/notes/notebooks/0-C3A40648AD0C9170!194485\",\"createdTime\":\"2015-06-15T14:48:32.357Z\",\"name\":\"Michelle's Lab Notebook\",\"createdBy\":\"Ansom Voodoo\",\"lastModifiedBy\":\"Michelle Tomczyk\",\"lastModifiedTime\":\"2018-04-09T20:16:56.763Z\",\"isDefault\":false,\"userRole\":\"Contributor\",\"isShared\":true,\"sectionsUrl\":\"https://www.onenote.com/api/v1.0/me/notes/notebooks/0-C3A40648AD0C9170!194485/sections\",\"sectionGroupsUrl\":\"https://www.onenote.com/api/v1.0/me/notes/notebooks/0-C3A40648AD0C9170!194485/sectionGroups\",\"links\":{\r\n        \"oneNoteClientUrl\":{\r\n          \"href\":\"onenote:https://d.docs.live.net/c3a40648ad0c9170/ansom/Expt.ansom/Personal%20Notebooks/Michelle's%20Lab%20Notebook\"\r\n        },\"oneNoteWebUrl\":{\r\n          \"href\":\"https://onedrive.live.com/redir.aspx?cid=c3a40648ad0c9170&page=edit&resid=C3A40648AD0C9170!194485&parId=C3A40648AD0C9170!131418\"\r\n        }\r\n      }\r\n    },{\r\n      \"id\":\"0-C3A40648AD0C9170!191750\",\"self\":\"https://www.onenote.com/api/v1.0/me/notes/notebooks/0-C3A40648AD0C9170!191750\",\"createdTime\":\"2014-03-22T19:48:56.117Z\",\"name\":\"MPMS-SQUID\",\"createdBy\":\"Ansom Voodoo\",\"lastModifiedBy\":\"Ansom Voodoo\",\"lastModifiedTime\":\"2018-04-09T20:16:56.763Z\",\"isDefault\":false,\"userRole\":\"Contributor\",\"isShared\":true,\"sectionsUrl\":\"https://www.onenote.com/api/v1.0/me/notes/notebooks/0-C3A40648AD0C9170!191750/sections\",\"sectionGroupsUrl\":\"https://www.onenote.com/api/v1.0/me/notes/notebooks/0-C3A40648AD0C9170!191750/sectionGroups\",\"links\":{\r\n        \"oneNoteClientUrl\":{\r\n          \"href\":\"onenote:https://d.docs.live.net/c3a40648ad0c9170/ansom/Expt.ansom/Experiment%20Notebooks/MPMS-SQUID\"\r\n        },\"oneNoteWebUrl\":{\r\n          \"href\":\"https://onedrive.live.com/redir.aspx?cid=c3a40648ad0c9170&page=edit&resid=C3A40648AD0C9170!191750&parId=C3A40648AD0C9170!131421\"\r\n        }\r\n      }\r\n    },{\r\n      \"id\":\"0-962DFAE583894FEA!194\",\"self\":\"https://www.onenote.com/api/v1.0/me/notes/notebooks/0-962DFAE583894FEA!194\",\"createdTime\":\"2017-07-06T01:32:00.127Z\",\"name\":\"My Notebook\",\"createdBy\":\"Joseph Albro\",\"lastModifiedBy\":\"Joseph Albro\",\"lastModifiedTime\":\"2018-04-05T03:37:14.07Z\",\"isDefault\":true,\"userRole\":\"Owner\",\"isShared\":false,\"sectionsUrl\":\"https://www.onenote.com/api/v1.0/me/notes/notebooks/0-962DFAE583894FEA!194/sections\",\"sectionGroupsUrl\":\"https://www.onenote.com/api/v1.0/me/notes/notebooks/0-962DFAE583894FEA!194/sectionGroups\",\"links\":{\r\n        \"oneNoteClientUrl\":{\r\n          \"href\":\"onenote:https://d.docs.live.net/962dfae583894fea/Documents/My%20Notebook\"\r\n        },\"oneNoteWebUrl\":{\r\n          \"href\":\"https://onedrive.live.com/redir.aspx?cid=962dfae583894fea&page=edit&resid=962DFAE583894FEA!194\"\r\n        }\r\n      }\r\n    },{\r\n      \"id\":\"0-962DFAE583894FEA!211\",\"self\":\"https://www.onenote.com/api/v1.0/me/notes/notebooks/0-962DFAE583894FEA!211\",\"createdTime\":\"2017-09-23T20:18:52.367Z\",\"name\":\"Nanosurf Easyscan 2\",\"createdBy\":\"Joseph Albro\",\"lastModifiedBy\":\"Joseph Albro\",\"lastModifiedTime\":\"2018-04-05T06:51:24.27Z\",\"isDefault\":false,\"userRole\":\"Owner\",\"isShared\":false,\"sectionsUrl\":\"https://www.onenote.com/api/v1.0/me/notes/notebooks/0-962DFAE583894FEA!211/sections\",\"sectionGroupsUrl\":\"https://www.onenote.com/api/v1.0/me/notes/notebooks/0-962DFAE583894FEA!211/sectionGroups\",\"links\":{\r\n        \"oneNoteClientUrl\":{\r\n          \"href\":\"onenote:https://d.docs.live.net/962dfae583894fea/Documents/Nanosurf%20Easyscan%202\"\r\n        },\"oneNoteWebUrl\":{\r\n          \"href\":\"https://onedrive.live.com/redir.aspx?cid=962dfae583894fea&page=edit&resid=962DFAE583894FEA!211\"\r\n        }\r\n      }\r\n    },{\r\n      \"id\":\"0-C3A40648AD0C9170!192178\",\"self\":\"https://www.onenote.com/api/v1.0/me/notes/notebooks/0-C3A40648AD0C9170!192178\",\"createdTime\":\"2014-08-08T16:03:08.453Z\",\"name\":\"New Notebook Name\",\"createdBy\":\"Ansom Voodoo\",\"lastModifiedBy\":\"Ansom Voodoo\",\"lastModifiedTime\":\"2018-04-09T20:16:56.763Z\",\"isDefault\":false,\"userRole\":\"Contributor\",\"isShared\":true,\"sectionsUrl\":\"https://www.onenote.com/api/v1.0/me/notes/notebooks/0-C3A40648AD0C9170!192178/sections\",\"sectionGroupsUrl\":\"https://www.onenote.com/api/v1.0/me/notes/notebooks/0-C3A40648AD0C9170!192178/sectionGroups\",\"links\":{\r\n        \"oneNoteClientUrl\":{\r\n          \"href\":\"onenote:https://d.docs.live.net/c3a40648ad0c9170/ansom/Documents/New%20Notebook%20Name\"\r\n        },\"oneNoteWebUrl\":{\r\n          \"href\":\"https://onedrive.live.com/redir.aspx?cid=c3a40648ad0c9170&page=edit&resid=C3A40648AD0C9170!192178&parId=C3A40648AD0C9170!106\"\r\n        }\r\n      }\r\n    },{\r\n      \"id\":\"0-C3A40648AD0C9170!193445\",\"self\":\"https://www.onenote.com/api/v1.0/me/notes/notebooks/0-C3A40648AD0C9170!193445\",\"createdTime\":\"2014-10-30T16:30:10.503Z\",\"name\":\"NHMFL March Notes\",\"createdBy\":\"Ansom Voodoo\",\"lastModifiedBy\":\"Megan Kirkendall\",\"lastModifiedTime\":\"2018-04-09T20:16:56.763Z\",\"isDefault\":false,\"userRole\":\"Contributor\",\"isShared\":true,\"sectionsUrl\":\"https://www.onenote.com/api/v1.0/me/notes/notebooks/0-C3A40648AD0C9170!193445/sections\",\"sectionGroupsUrl\":\"https://www.onenote.com/api/v1.0/me/notes/notebooks/0-C3A40648AD0C9170!193445/sectionGroups\",\"links\":{\r\n        \"oneNoteClientUrl\":{\r\n          \"href\":\"onenote:https://d.docs.live.net/c3a40648ad0c9170/ansom/Expt.ansom/Experiment%20Notebooks/NHMFL/NHMFL%20March%20Notes\"\r\n        },\"oneNoteWebUrl\":{\r\n          \"href\":\"https://onedrive.live.com/redir.aspx?cid=c3a40648ad0c9170&page=edit&resid=C3A40648AD0C9170!193445&parId=C3A40648AD0C9170!191626\"\r\n        }\r\n      }\r\n    },{\r\n      \"id\":\"0-C3A40648AD0C9170!191873\",\"self\":\"https://www.onenote.com/api/v1.0/me/notes/notebooks/0-C3A40648AD0C9170!191873\",\"createdTime\":\"2014-05-05T15:19:17.383Z\",\"name\":\"Nicholas's Lab Notebook\",\"createdBy\":\"Ansom Voodoo\",\"lastModifiedBy\":\"Yuhe Tang\",\"lastModifiedTime\":\"2018-04-09T20:16:56.763Z\",\"isDefault\":false,\"userRole\":\"Contributor\",\"isShared\":true,\"sectionsUrl\":\"https://www.onenote.com/api/v1.0/me/notes/notebooks/0-C3A40648AD0C9170!191873/sections\",\"sectionGroupsUrl\":\"https://www.onenote.com/api/v1.0/me/notes/notebooks/0-C3A40648AD0C9170!191873/sectionGroups\",\"links\":{\r\n        \"oneNoteClientUrl\":{\r\n          \"href\":\"onenote:https://d.docs.live.net/c3a40648ad0c9170/ansom/Expt.ansom/Personal%20Notebooks/Alumni/Nicholas's%20Lab%20Notebook\"\r\n        },\"oneNoteWebUrl\":{\r\n          \"href\":\"https://onedrive.live.com/redir.aspx?cid=c3a40648ad0c9170&page=edit&resid=C3A40648AD0C9170!191873&parId=C3A40648AD0C9170!194471\"\r\n        }\r\n      }\r\n    },{\r\n      \"id\":\"0-C3A40648AD0C9170!2629\",\"self\":\"https://www.onenote.com/api/v1.0/me/notes/notebooks/0-C3A40648AD0C9170!2629\",\"createdTime\":\"2013-06-03T19:38:30Z\",\"name\":\"Notes\",\"createdBy\":\"Ansom Voodoo\",\"lastModifiedBy\":\"Guanglei Cheng\",\"lastModifiedTime\":\"2018-04-09T20:16:56.763Z\",\"isDefault\":false,\"userRole\":\"Contributor\",\"isShared\":true,\"sectionsUrl\":\"https://www.onenote.com/api/v1.0/me/notes/notebooks/0-C3A40648AD0C9170!2629/sections\",\"sectionGroupsUrl\":\"https://www.onenote.com/api/v1.0/me/notes/notebooks/0-C3A40648AD0C9170!2629/sectionGroups\",\"links\":{\r\n        \"oneNoteClientUrl\":{\r\n          \"href\":\"onenote:https://d.docs.live.net/c3a40648ad0c9170/ansom/Manuscripts.ansom/ZZZ%20Old/Confined%20wire/ms/Notes\"\r\n        },\"oneNoteWebUrl\":{\r\n          \"href\":\"https://onedrive.live.com/redir.aspx?cid=c3a40648ad0c9170&page=edit&resid=C3A40648AD0C9170!2629&parId=C3A40648AD0C9170!2609\"\r\n        }\r\n      }\r\n    },{\r\n      \"id\":\"0-C3A40648AD0C9170!613\",\"self\":\"https://www.onenote.com/api/v1.0/me/notes/notebooks/0-C3A40648AD0C9170!613\",\"createdTime\":\"2012-10-11T14:03:51.773Z\",\"name\":\"Oxford DR200\",\"createdBy\":\"Ansom Voodoo\",\"lastModifiedBy\":\"Megan Kirkendall\",\"lastModifiedTime\":\"2018-04-09T20:16:56.763Z\",\"isDefault\":false,\"userRole\":\"Contributor\",\"isShared\":true,\"sectionsUrl\":\"https://www.onenote.com/api/v1.0/me/notes/notebooks/0-C3A40648AD0C9170!613/sections\",\"sectionGroupsUrl\":\"https://www.onenote.com/api/v1.0/me/notes/notebooks/0-C3A40648AD0C9170!613/sectionGroups\",\"links\":{\r\n        \"oneNoteClientUrl\":{\r\n          \"href\":\"onenote:https://d.docs.live.net/c3a40648ad0c9170/ansom/Expt.ansom/Instrument%20Notebooks/Oxford%20DR200\"\r\n        },\"oneNoteWebUrl\":{\r\n          \"href\":\"https://onedrive.live.com/redir.aspx?cid=c3a40648ad0c9170&page=edit&resid=C3A40648AD0C9170!613&parId=C3A40648AD0C9170!72393\"\r\n        }\r\n      }\r\n    },{\r\n      \"id\":\"0-C3A40648AD0C9170!191936\",\"self\":\"https://www.onenote.com/api/v1.0/me/notes/notebooks/0-C3A40648AD0C9170!191936\",\"createdTime\":\"2014-06-06T18:07:06.19Z\",\"name\":\"Pai's Lab Notebook\",\"createdBy\":\"Ansom Voodoo\",\"lastModifiedBy\":\"Yun-Yi Pai\",\"lastModifiedTime\":\"2018-04-09T20:16:56.763Z\",\"isDefault\":false,\"userRole\":\"Contributor\",\"isShared\":true,\"sectionsUrl\":\"https://www.onenote.com/api/v1.0/me/notes/notebooks/0-C3A40648AD0C9170!191936/sections\",\"sectionGroupsUrl\":\"https://www.onenote.com/api/v1.0/me/notes/notebooks/0-C3A40648AD0C9170!191936/sectionGroups\",\"links\":{\r\n        \"oneNoteClientUrl\":{\r\n          \"href\":\"onenote:https://d.docs.live.net/c3a40648ad0c9170/ansom/Expt.ansom/Personal%20Notebooks/Pai's%20Lab%20Notebook\"\r\n        },\"oneNoteWebUrl\":{\r\n          \"href\":\"https://onedrive.live.com/redir.aspx?cid=c3a40648ad0c9170&page=edit&resid=C3A40648AD0C9170!191936&parId=C3A40648AD0C9170!131418\"\r\n        }\r\n      }\r\n    },{\r\n      \"id\":\"0-C3A40648AD0C9170!217831\",\"self\":\"https://www.onenote.com/api/v1.0/me/notes/notebooks/0-C3A40648AD0C9170!217831\",\"createdTime\":\"2016-12-09T19:41:25.47Z\",\"name\":\"Pai's Lab Notebook\",\"createdBy\":\"Ansom Voodoo\",\"lastModifiedBy\":\"Ansom Voodoo\",\"lastModifiedTime\":\"2017-09-28T15:01:37.08Z\",\"isDefault\":false,\"userRole\":\"Contributor\",\"isShared\":true,\"sectionsUrl\":\"https://www.onenote.com/api/v1.0/me/notes/notebooks/0-C3A40648AD0C9170!217831/sections\",\"sectionGroupsUrl\":\"https://www.onenote.com/api/v1.0/me/notes/notebooks/0-C3A40648AD0C9170!217831/sectionGroups\",\"links\":{\r\n        \"oneNoteClientUrl\":{\r\n          \"href\":\"onenote:https://d.docs.live.net/c3a40648ad0c9170/ansom/Expt.ansom/Personal%20Notebooks/Temp/Pai's%20Lab%20Notebook\"\r\n        },\"oneNoteWebUrl\":{\r\n          \"href\":\"https://onedrive.live.com/redir.aspx?cid=c3a40648ad0c9170&page=edit&resid=C3A40648AD0C9170!217831&parId=C3A40648AD0C9170!217105\"\r\n        }\r\n      }\r\n    },{\r\n      \"id\":\"0-C3A40648AD0C9170!191602\",\"self\":\"https://www.onenote.com/api/v1.0/me/notes/notebooks/0-C3A40648AD0C9170!191602\",\"createdTime\":\"2014-01-15T14:46:10.727Z\",\"name\":\"Patent for controlled magnetism on LAOSTO\",\"createdBy\":\"Ansom Voodoo\",\"lastModifiedBy\":\"Feng Bi\",\"lastModifiedTime\":\"2018-04-09T20:16:56.763Z\",\"isDefault\":false,\"userRole\":\"Contributor\",\"isShared\":true,\"sectionsUrl\":\"https://www.onenote.com/api/v1.0/me/notes/notebooks/0-C3A40648AD0C9170!191602/sections\",\"sectionGroupsUrl\":\"https://www.onenote.com/api/v1.0/me/notes/notebooks/0-C3A40648AD0C9170!191602/sectionGroups\",\"links\":{\r\n        \"oneNoteClientUrl\":{\r\n          \"href\":\"onenote:https://d.docs.live.net/c3a40648ad0c9170/ansom/Manuscripts.ansom/Patent%20application/Patent%20for%20controlled%20magnetism%20on%20LAOSTO\"\r\n        },\"oneNoteWebUrl\":{\r\n          \"href\":\"https://onedrive.live.com/redir.aspx?cid=c3a40648ad0c9170&page=edit&resid=C3A40648AD0C9170!191602&parId=C3A40648AD0C9170!191598\"\r\n        }\r\n      }\r\n    },{\r\n      \"id\":\"0-C3A40648AD0C9170!148588\",\"self\":\"https://www.onenote.com/api/v1.0/me/notes/notebooks/0-C3A40648AD0C9170!148588\",\"createdTime\":\"2013-10-31T10:21:51.637Z\",\"name\":\"Patrick's Lab Notebook\",\"createdBy\":\"Ansom Voodoo\",\"lastModifiedBy\":\"Patrick Irvin\",\"lastModifiedTime\":\"2018-04-09T20:16:56.763Z\",\"isDefault\":false,\"userRole\":\"Contributor\",\"isShared\":true,\"sectionsUrl\":\"https://www.onenote.com/api/v1.0/me/notes/notebooks/0-C3A40648AD0C9170!148588/sections\",\"sectionGroupsUrl\":\"https://www.onenote.com/api/v1.0/me/notes/notebooks/0-C3A40648AD0C9170!148588/sectionGroups\",\"links\":{\r\n        \"oneNoteClientUrl\":{\r\n          \"href\":\"onenote:https://d.docs.live.net/c3a40648ad0c9170/ansom/Expt.ansom/Personal%20Notebooks/Patrick's%20Lab%20Notebook\"\r\n        },\"oneNoteWebUrl\":{\r\n          \"href\":\"https://onedrive.live.com/redir.aspx?cid=c3a40648ad0c9170&page=edit&resid=C3A40648AD0C9170!148588&parId=C3A40648AD0C9170!131418\"\r\n        }\r\n      }\r\n    },{\r\n      \"id\":\"0-C3A40648AD0C9170!133\",\"self\":\"https://www.onenote.com/api/v1.0/me/notes/notebooks/0-C3A40648AD0C9170!133\",\"createdTime\":\"2012-04-21T03:26:16.263Z\",\"name\":\"Personal (Web)\",\"createdBy\":\"Ansom Voodoo\",\"lastModifiedBy\":\"Ansom Voodoo\",\"lastModifiedTime\":\"2018-04-10T21:38:22.477Z\",\"isDefault\":false,\"userRole\":\"Contributor\",\"isShared\":true,\"sectionsUrl\":\"https://www.onenote.com/api/v1.0/me/notes/notebooks/0-C3A40648AD0C9170!133/sections\",\"sectionGroupsUrl\":\"https://www.onenote.com/api/v1.0/me/notes/notebooks/0-C3A40648AD0C9170!133/sectionGroups\",\"links\":{\r\n        \"oneNoteClientUrl\":{\r\n          \"href\":\"onenote:https://d.docs.live.net/c3a40648ad0c9170/ansom/Documents/Personal%20(Web)\"\r\n        },\"oneNoteWebUrl\":{\r\n          \"href\":\"https://onedrive.live.com/redir.aspx?cid=c3a40648ad0c9170&page=edit&resid=C3A40648AD0C9170!133&parId=C3A40648AD0C9170!106\"\r\n        }\r\n      }\r\n    },{\r\n      \"id\":\"0-C3A40648AD0C9170!191905\",\"self\":\"https://www.onenote.com/api/v1.0/me/notes/notebooks/0-C3A40648AD0C9170!191905\",\"createdTime\":\"2014-05-22T15:38:24.987Z\",\"name\":\"PPMS 2\",\"createdBy\":\"Ansom Voodoo\",\"lastModifiedBy\":\"Ansom Voodoo\",\"lastModifiedTime\":\"2018-04-09T20:16:56.763Z\",\"isDefault\":false,\"userRole\":\"Contributor\",\"isShared\":true,\"sectionsUrl\":\"https://www.onenote.com/api/v1.0/me/notes/notebooks/0-C3A40648AD0C9170!191905/sections\",\"sectionGroupsUrl\":\"https://www.onenote.com/api/v1.0/me/notes/notebooks/0-C3A40648AD0C9170!191905/sectionGroups\",\"links\":{\r\n        \"oneNoteClientUrl\":{\r\n          \"href\":\"onenote:https://d.docs.live.net/c3a40648ad0c9170/ansom/Expt.ansom/Instrument%20Notebooks/PPMS%202\"\r\n        },\"oneNoteWebUrl\":{\r\n          \"href\":\"https://onedrive.live.com/redir.aspx?cid=c3a40648ad0c9170&page=edit&resid=C3A40648AD0C9170!191905&parId=C3A40648AD0C9170!72393\"\r\n        }\r\n      }\r\n    },{\r\n      \"id\":\"0-C3A40648AD0C9170!192044\",\"self\":\"https://www.onenote.com/api/v1.0/me/notes/notebooks/0-C3A40648AD0C9170!192044\",\"createdTime\":\"2014-07-03T13:19:12.377Z\",\"name\":\"PPMS key results presentation\",\"createdBy\":\"Ansom Voodoo\",\"lastModifiedBy\":\"Ansom Voodoo\",\"lastModifiedTime\":\"2018-04-09T20:16:56.763Z\",\"isDefault\":false,\"userRole\":\"Contributor\",\"isShared\":true,\"sectionsUrl\":\"https://www.onenote.com/api/v1.0/me/notes/notebooks/0-C3A40648AD0C9170!192044/sections\",\"sectionGroupsUrl\":\"https://www.onenote.com/api/v1.0/me/notes/notebooks/0-C3A40648AD0C9170!192044/sectionGroups\",\"links\":{\r\n        \"oneNoteClientUrl\":{\r\n          \"href\":\"onenote:https://d.docs.live.net/c3a40648ad0c9170/ansom/Expt.ansom/Experiment%20Notebooks/PPMS%20key%20results%20presentation\"\r\n        },\"oneNoteWebUrl\":{\r\n          \"href\":\"https://onedrive.live.com/redir.aspx?cid=c3a40648ad0c9170&page=edit&resid=C3A40648AD0C9170!192044&parId=C3A40648AD0C9170!131421\"\r\n        }\r\n      }\r\n    },{\r\n      \"id\":\"0-C3A40648AD0C9170!195833\",\"self\":\"https://www.onenote.com/api/v1.0/me/notes/notebooks/0-C3A40648AD0C9170!195833\",\"createdTime\":\"2015-11-20T22:48:31.573Z\",\"name\":\"PPMS(OLD)\",\"createdBy\":\"Ansom Voodoo\",\"lastModifiedBy\":\"Ansom Voodoo\",\"lastModifiedTime\":\"2018-04-09T20:16:56.763Z\",\"isDefault\":false,\"userRole\":\"Contributor\",\"isShared\":true,\"sectionsUrl\":\"https://www.onenote.com/api/v1.0/me/notes/notebooks/0-C3A40648AD0C9170!195833/sections\",\"sectionGroupsUrl\":\"https://www.onenote.com/api/v1.0/me/notes/notebooks/0-C3A40648AD0C9170!195833/sectionGroups\",\"links\":{\r\n        \"oneNoteClientUrl\":{\r\n          \"href\":\"onenote:https://d.docs.live.net/c3a40648ad0c9170/ansom/Documents/PPMS(OLD)\"\r\n        },\"oneNoteWebUrl\":{\r\n          \"href\":\"https://onedrive.live.com/redir.aspx?cid=c3a40648ad0c9170&page=edit&resid=C3A40648AD0C9170!195833&parId=C3A40648AD0C9170!106\"\r\n        }\r\n      }\r\n    },{\r\n      \"id\":\"0-C3A40648AD0C9170!195927\",\"self\":\"https://www.onenote.com/api/v1.0/me/notes/notebooks/0-C3A40648AD0C9170!195927\",\"createdTime\":\"2015-11-24T21:50:22.12Z\",\"name\":\"PPMSNEW\",\"createdBy\":\"Ansom Voodoo\",\"lastModifiedBy\":\"Michelle Tomczyk\",\"lastModifiedTime\":\"2018-04-10T22:35:54.987Z\",\"isDefault\":false,\"userRole\":\"Contributor\",\"isShared\":true,\"sectionsUrl\":\"https://www.onenote.com/api/v1.0/me/notes/notebooks/0-C3A40648AD0C9170!195927/sections\",\"sectionGroupsUrl\":\"https://www.onenote.com/api/v1.0/me/notes/notebooks/0-C3A40648AD0C9170!195927/sectionGroups\",\"links\":{\r\n        \"oneNoteClientUrl\":{\r\n          \"href\":\"onenote:https://d.docs.live.net/c3a40648ad0c9170/ansom/Expt.ansom/Instrument%20Notebooks/PPMSNEW\"\r\n        },\"oneNoteWebUrl\":{\r\n          \"href\":\"https://onedrive.live.com/redir.aspx?cid=c3a40648ad0c9170&page=edit&resid=C3A40648AD0C9170!195927&parId=C3A40648AD0C9170!72393\"\r\n        }\r\n      }\r\n    },{\r\n      \"id\":\"0-C3A40648AD0C9170!195062\",\"self\":\"https://www.onenote.com/api/v1.0/me/notes/notebooks/0-C3A40648AD0C9170!195062\",\"createdTime\":\"2015-09-14T13:45:06.457Z\",\"name\":\"Project Discussion Summary\",\"createdBy\":\"Ansom Voodoo\",\"lastModifiedBy\":\"Ansom Voodoo\",\"lastModifiedTime\":\"2018-04-09T20:16:56.763Z\",\"isDefault\":false,\"userRole\":\"Contributor\",\"isShared\":true,\"sectionsUrl\":\"https://www.onenote.com/api/v1.0/me/notes/notebooks/0-C3A40648AD0C9170!195062/sections\",\"sectionGroupsUrl\":\"https://www.onenote.com/api/v1.0/me/notes/notebooks/0-C3A40648AD0C9170!195062/sectionGroups\",\"links\":{\r\n        \"oneNoteClientUrl\":{\r\n          \"href\":\"onenote:https://d.docs.live.net/c3a40648ad0c9170/ansom/Documents/Project%20Discussion%20Summary\"\r\n        },\"oneNoteWebUrl\":{\r\n          \"href\":\"https://onedrive.live.com/redir.aspx?cid=c3a40648ad0c9170&page=edit&resid=C3A40648AD0C9170!195062&parId=C3A40648AD0C9170!106\"\r\n        }\r\n      }\r\n    },{\r\n      \"id\":\"0-C3A40648AD0C9170!216298\",\"self\":\"https://www.onenote.com/api/v1.0/me/notes/notebooks/0-C3A40648AD0C9170!216298\",\"createdTime\":\"2016-07-08T20:50:55.157Z\",\"name\":\"Qi Zhang\",\"createdBy\":\"Ansom Voodoo\",\"lastModifiedBy\":\"\",\"lastModifiedTime\":\"2018-04-09T20:16:56.763Z\",\"isDefault\":false,\"userRole\":\"Contributor\",\"isShared\":true,\"sectionsUrl\":\"https://www.onenote.com/api/v1.0/me/notes/notebooks/0-C3A40648AD0C9170!216298/sections\",\"sectionGroupsUrl\":\"https://www.onenote.com/api/v1.0/me/notes/notebooks/0-C3A40648AD0C9170!216298/sectionGroups\",\"links\":{\r\n        \"oneNoteClientUrl\":{\r\n          \"href\":\"onenote:https://d.docs.live.net/c3a40648ad0c9170/ansom/Expt.ansom/Personal%20Notebooks/Qi%20Zhang\"\r\n        },\"oneNoteWebUrl\":{\r\n          \"href\":\"https://onedrive.live.com/redir.aspx?cid=c3a40648ad0c9170&page=edit&resid=C3A40648AD0C9170!216298&parId=C3A40648AD0C9170!131418\"\r\n        }\r\n      }\r\n    },{\r\n      \"id\":\"0-C3A40648AD0C9170!191970\",\"self\":\"https://www.onenote.com/api/v1.0/me/notes/notebooks/0-C3A40648AD0C9170!191970\",\"createdTime\":\"2014-06-11T17:34:27.893Z\",\"name\":\"Qing Guo's Lab Notebook\",\"createdBy\":\"Ansom Voodoo\",\"lastModifiedBy\":\"Ansom Voodoo\",\"lastModifiedTime\":\"2018-04-09T20:16:56.763Z\",\"isDefault\":false,\"userRole\":\"Contributor\",\"isShared\":true,\"sectionsUrl\":\"https://www.onenote.com/api/v1.0/me/notes/notebooks/0-C3A40648AD0C9170!191970/sections\",\"sectionGroupsUrl\":\"https://www.onenote.com/api/v1.0/me/notes/notebooks/0-C3A40648AD0C9170!191970/sectionGroups\",\"links\":{\r\n        \"oneNoteClientUrl\":{\r\n          \"href\":\"onenote:https://d.docs.live.net/c3a40648ad0c9170/ansom/Expt.ansom/Personal%20Notebooks/Qing%20Guo's%20Lab%20Notebook\"\r\n        },\"oneNoteWebUrl\":{\r\n          \"href\":\"https://onedrive.live.com/redir.aspx?cid=c3a40648ad0c9170&page=edit&resid=C3A40648AD0C9170!191970&parId=C3A40648AD0C9170!131418\"\r\n        }\r\n      }\r\n    },{\r\n      \"id\":\"0-C3A40648AD0C9170!197971\",\"self\":\"https://www.onenote.com/api/v1.0/me/notes/notebooks/0-C3A40648AD0C9170!197971\",\"createdTime\":\"2016-05-08T16:02:07.747Z\",\"name\":\"Samples\",\"createdBy\":\"Ansom Voodoo\",\"lastModifiedBy\":\"Ansom Voodoo\",\"lastModifiedTime\":\"2018-04-10T19:15:07.61Z\",\"isDefault\":false,\"userRole\":\"Contributor\",\"isShared\":true,\"sectionsUrl\":\"https://www.onenote.com/api/v1.0/me/notes/notebooks/0-C3A40648AD0C9170!197971/sections\",\"sectionGroupsUrl\":\"https://www.onenote.com/api/v1.0/me/notes/notebooks/0-C3A40648AD0C9170!197971/sectionGroups\",\"links\":{\r\n        \"oneNoteClientUrl\":{\r\n          \"href\":\"onenote:https://d.docs.live.net/c3a40648ad0c9170/ansom/Expt.ansom/Instrument%20Notebooks/Samples\"\r\n        },\"oneNoteWebUrl\":{\r\n          \"href\":\"https://onedrive.live.com/redir.aspx?cid=c3a40648ad0c9170&page=edit&resid=C3A40648AD0C9170!197971&parId=C3A40648AD0C9170!72393\"\r\n        }\r\n      }\r\n    },{\r\n      \"id\":\"0-C3A40648AD0C9170!160781\",\"self\":\"https://www.onenote.com/api/v1.0/me/notes/notebooks/0-C3A40648AD0C9170!160781\",\"createdTime\":\"2013-11-01T19:47:22.48Z\",\"name\":\"THz1\",\"createdBy\":\"Ansom Voodoo\",\"lastModifiedBy\":\"Lu Chen\",\"lastModifiedTime\":\"2018-04-10T18:10:03.273Z\",\"isDefault\":false,\"userRole\":\"Contributor\",\"isShared\":true,\"sectionsUrl\":\"https://www.onenote.com/api/v1.0/me/notes/notebooks/0-C3A40648AD0C9170!160781/sections\",\"sectionGroupsUrl\":\"https://www.onenote.com/api/v1.0/me/notes/notebooks/0-C3A40648AD0C9170!160781/sectionGroups\",\"links\":{\r\n        \"oneNoteClientUrl\":{\r\n          \"href\":\"onenote:https://d.docs.live.net/c3a40648ad0c9170/ansom/Expt.ansom/Instrument%20Notebooks/THz1\"\r\n        },\"oneNoteWebUrl\":{\r\n          \"href\":\"https://onedrive.live.com/redir.aspx?cid=c3a40648ad0c9170&page=edit&resid=C3A40648AD0C9170!160781&parId=C3A40648AD0C9170!72393\"\r\n        }\r\n      }\r\n    },{\r\n      \"id\":\"0-C3A40648AD0C9170!191924\",\"self\":\"https://www.onenote.com/api/v1.0/me/notes/notebooks/0-C3A40648AD0C9170!191924\",\"createdTime\":\"2014-06-02T20:54:55.547Z\",\"name\":\"VO2 Experiments\",\"createdBy\":\"Ansom Voodoo\",\"lastModifiedBy\":\"Ansom Voodoo\",\"lastModifiedTime\":\"2018-04-09T20:16:56.763Z\",\"isDefault\":false,\"userRole\":\"Contributor\",\"isShared\":true,\"sectionsUrl\":\"https://www.onenote.com/api/v1.0/me/notes/notebooks/0-C3A40648AD0C9170!191924/sections\",\"sectionGroupsUrl\":\"https://www.onenote.com/api/v1.0/me/notes/notebooks/0-C3A40648AD0C9170!191924/sectionGroups\",\"links\":{\r\n        \"oneNoteClientUrl\":{\r\n          \"href\":\"onenote:https://d.docs.live.net/c3a40648ad0c9170/ansom/Documents/VO2%20Experiments\"\r\n        },\"oneNoteWebUrl\":{\r\n          \"href\":\"https://onedrive.live.com/redir.aspx?cid=c3a40648ad0c9170&page=edit&resid=C3A40648AD0C9170!191924&parId=C3A40648AD0C9170!106\"\r\n        }\r\n      }\r\n    },{\r\n      \"id\":\"0-C3A40648AD0C9170!191957\",\"self\":\"https://www.onenote.com/api/v1.0/me/notes/notebooks/0-C3A40648AD0C9170!191957\",\"createdTime\":\"2014-06-10T15:13:38.41Z\",\"name\":\"VO2 Experimetns\",\"createdBy\":\"Ansom Voodoo\",\"lastModifiedBy\":\"Ansom Voodoo\",\"lastModifiedTime\":\"2018-04-09T20:16:56.763Z\",\"isDefault\":false,\"userRole\":\"Contributor\",\"isShared\":true,\"sectionsUrl\":\"https://www.onenote.com/api/v1.0/me/notes/notebooks/0-C3A40648AD0C9170!191957/sections\",\"sectionGroupsUrl\":\"https://www.onenote.com/api/v1.0/me/notes/notebooks/0-C3A40648AD0C9170!191957/sectionGroups\",\"links\":{\r\n        \"oneNoteClientUrl\":{\r\n          \"href\":\"onenote:https://d.docs.live.net/c3a40648ad0c9170/ansom/Documents/VO2%20Experimetns\"\r\n        },\"oneNoteWebUrl\":{\r\n          \"href\":\"https://onedrive.live.com/redir.aspx?cid=c3a40648ad0c9170&page=edit&resid=C3A40648AD0C9170!191957&parId=C3A40648AD0C9170!106\"\r\n        }\r\n      }\r\n    },{\r\n      \"id\":\"0-C3A40648AD0C9170!191512\",\"self\":\"https://www.onenote.com/api/v1.0/me/notes/notebooks/0-C3A40648AD0C9170!191512\",\"createdTime\":\"2014-01-08T19:34:49.92Z\",\"name\":\"Wirebonder\",\"createdBy\":\"Ansom Voodoo\",\"lastModifiedBy\":\"Ansom Voodoo\",\"lastModifiedTime\":\"2018-04-09T20:16:56.763Z\",\"isDefault\":false,\"userRole\":\"Contributor\",\"isShared\":true,\"sectionsUrl\":\"https://www.onenote.com/api/v1.0/me/notes/notebooks/0-C3A40648AD0C9170!191512/sections\",\"sectionGroupsUrl\":\"https://www.onenote.com/api/v1.0/me/notes/notebooks/0-C3A40648AD0C9170!191512/sectionGroups\",\"links\":{\r\n        \"oneNoteClientUrl\":{\r\n          \"href\":\"onenote:https://d.docs.live.net/c3a40648ad0c9170/ansom/Expt.ansom/Instrument%20Notebooks/Wirebonder\"\r\n        },\"oneNoteWebUrl\":{\r\n          \"href\":\"https://onedrive.live.com/redir.aspx?cid=c3a40648ad0c9170&page=edit&resid=C3A40648AD0C9170!191512&parId=C3A40648AD0C9170!72393\"\r\n        }\r\n      }\r\n    },{\r\n      \"id\":\"0-C3A40648AD0C9170!197386\",\"self\":\"https://www.onenote.com/api/v1.0/me/notes/notebooks/0-C3A40648AD0C9170!197386\",\"createdTime\":\"2016-04-12T14:53:13.4Z\",\"name\":\"Wisconsin LAOSTO\",\"createdBy\":\"Ansom Voodoo\",\"lastModifiedBy\":\"Ansom Voodoo\",\"lastModifiedTime\":\"2018-04-09T20:16:56.763Z\",\"isDefault\":false,\"userRole\":\"Contributor\",\"isShared\":true,\"sectionsUrl\":\"https://www.onenote.com/api/v1.0/me/notes/notebooks/0-C3A40648AD0C9170!197386/sections\",\"sectionGroupsUrl\":\"https://www.onenote.com/api/v1.0/me/notes/notebooks/0-C3A40648AD0C9170!197386/sectionGroups\",\"links\":{\r\n        \"oneNoteClientUrl\":{\r\n          \"href\":\"onenote:https://d.docs.live.net/c3a40648ad0c9170/ansom/Documents/Wisconsin%20LAOSTO\"\r\n        },\"oneNoteWebUrl\":{\r\n          \"href\":\"https://onedrive.live.com/redir.aspx?cid=c3a40648ad0c9170&page=edit&resid=C3A40648AD0C9170!197386&parId=C3A40648AD0C9170!106\"\r\n        }\r\n      }\r\n    },{\r\n      \"id\":\"0-C3A40648AD0C9170!216909\",\"self\":\"https://www.onenote.com/api/v1.0/me/notes/notebooks/0-C3A40648AD0C9170!216909\",\"createdTime\":\"2016-08-29T18:36:16.753Z\",\"name\":\"Xinyi Wu's Lab Notebook\",\"createdBy\":\"Ansom Voodoo\",\"lastModifiedBy\":\"\",\"lastModifiedTime\":\"2018-04-09T20:16:56.763Z\",\"isDefault\":false,\"userRole\":\"Contributor\",\"isShared\":true,\"sectionsUrl\":\"https://www.onenote.com/api/v1.0/me/notes/notebooks/0-C3A40648AD0C9170!216909/sections\",\"sectionGroupsUrl\":\"https://www.onenote.com/api/v1.0/me/notes/notebooks/0-C3A40648AD0C9170!216909/sectionGroups\",\"links\":{\r\n        \"oneNoteClientUrl\":{\r\n          \"href\":\"onenote:https://d.docs.live.net/c3a40648ad0c9170/ansom/Expt.ansom/Personal%20Notebooks/Xinyi%20Wu's%20Lab%20Notebook\"\r\n        },\"oneNoteWebUrl\":{\r\n          \"href\":\"https://onedrive.live.com/redir.aspx?cid=c3a40648ad0c9170&page=edit&resid=C3A40648AD0C9170!216909&parId=C3A40648AD0C9170!131418\"\r\n        }\r\n      }\r\n    },{\r\n      \"id\":\"0-C3A40648AD0C9170!272758\",\"self\":\"https://www.onenote.com/api/v1.0/me/notes/notebooks/0-C3A40648AD0C9170!272758\",\"createdTime\":\"2017-10-12T23:26:26.893Z\",\"name\":\"Yang Hu's Labnotes\",\"createdBy\":\"Ansom Voodoo\",\"lastModifiedBy\":\"Ansom Voodoo\",\"lastModifiedTime\":\"2017-12-15T16:14:47.65Z\",\"isDefault\":false,\"userRole\":\"Contributor\",\"isShared\":true,\"sectionsUrl\":\"https://www.onenote.com/api/v1.0/me/notes/notebooks/0-C3A40648AD0C9170!272758/sections\",\"sectionGroupsUrl\":\"https://www.onenote.com/api/v1.0/me/notes/notebooks/0-C3A40648AD0C9170!272758/sectionGroups\",\"links\":{\r\n        \"oneNoteClientUrl\":{\r\n          \"href\":\"onenote:https://d.docs.live.net/c3a40648ad0c9170/ansom/Documents/Yang%20Hu's%20Labnotes\"\r\n        },\"oneNoteWebUrl\":{\r\n          \"href\":\"https://onedrive.live.com/redir.aspx?cid=c3a40648ad0c9170&page=edit&resid=C3A40648AD0C9170!272758&parId=C3A40648AD0C9170!106\"\r\n        }\r\n      }\r\n    },{\r\n      \"id\":\"0-C3A40648AD0C9170!271583\",\"self\":\"https://www.onenote.com/api/v1.0/me/notes/notebooks/0-C3A40648AD0C9170!271583\",\"createdTime\":\"2017-06-26T13:52:37.473Z\",\"name\":\"Yang Hu's Notebook\",\"createdBy\":\"Ansom Voodoo\",\"lastModifiedBy\":\"Ansom Voodoo\",\"lastModifiedTime\":\"2018-03-16T19:05:42.68Z\",\"isDefault\":false,\"userRole\":\"Contributor\",\"isShared\":true,\"sectionsUrl\":\"https://www.onenote.com/api/v1.0/me/notes/notebooks/0-C3A40648AD0C9170!271583/sections\",\"sectionGroupsUrl\":\"https://www.onenote.com/api/v1.0/me/notes/notebooks/0-C3A40648AD0C9170!271583/sectionGroups\",\"links\":{\r\n        \"oneNoteClientUrl\":{\r\n          \"href\":\"onenote:https://d.docs.live.net/c3a40648ad0c9170/ansom/Documents/Yang%20Hu's%20Notebook\"\r\n        },\"oneNoteWebUrl\":{\r\n          \"href\":\"https://onedrive.live.com/redir.aspx?cid=c3a40648ad0c9170&page=edit&resid=C3A40648AD0C9170!271583&parId=C3A40648AD0C9170!106\"\r\n        }\r\n      }\r\n    },{\r\n      \"id\":\"0-C3A40648AD0C9170!194465\",\"self\":\"https://www.onenote.com/api/v1.0/me/notes/notebooks/0-C3A40648AD0C9170!194465\",\"createdTime\":\"2015-06-11T14:01:46.307Z\",\"name\":\"Yuhe's lab Notebook\",\"createdBy\":\"Ansom Voodoo\",\"lastModifiedBy\":\"Yuhe Tang\",\"lastModifiedTime\":\"2018-04-10T21:38:30.027Z\",\"isDefault\":false,\"userRole\":\"Contributor\",\"isShared\":true,\"sectionsUrl\":\"https://www.onenote.com/api/v1.0/me/notes/notebooks/0-C3A40648AD0C9170!194465/sections\",\"sectionGroupsUrl\":\"https://www.onenote.com/api/v1.0/me/notes/notebooks/0-C3A40648AD0C9170!194465/sectionGroups\",\"links\":{\r\n        \"oneNoteClientUrl\":{\r\n          \"href\":\"onenote:https://d.docs.live.net/c3a40648ad0c9170/ansom/Expt.ansom/Personal%20Notebooks/Yuhe's%20lab%20Notebook\"\r\n        },\"oneNoteWebUrl\":{\r\n          \"href\":\"https://onedrive.live.com/redir.aspx?cid=c3a40648ad0c9170&page=edit&resid=C3A40648AD0C9170!194465&parId=C3A40648AD0C9170!131418\"\r\n        }\r\n      }\r\n    },{\r\n      \"id\":\"0-C3A40648AD0C9170!194479\",\"self\":\"https://www.onenote.com/api/v1.0/me/notes/notebooks/0-C3A40648AD0C9170!194479\",\"createdTime\":\"2015-06-13T18:32:27.067Z\",\"name\":\"Yuhe's Lab Notebook\",\"createdBy\":\"Ansom Voodoo\",\"lastModifiedBy\":\"Ansom Voodoo\",\"lastModifiedTime\":\"2018-04-09T20:16:56.763Z\",\"isDefault\":false,\"userRole\":\"Contributor\",\"isShared\":true,\"sectionsUrl\":\"https://www.onenote.com/api/v1.0/me/notes/notebooks/0-C3A40648AD0C9170!194479/sections\",\"sectionGroupsUrl\":\"https://www.onenote.com/api/v1.0/me/notes/notebooks/0-C3A40648AD0C9170!194479/sectionGroups\",\"links\":{\r\n        \"oneNoteClientUrl\":{\r\n          \"href\":\"onenote:https://d.docs.live.net/c3a40648ad0c9170/ansom/Documents/Yuhe's%20Lab%20Notebook\"\r\n        },\"oneNoteWebUrl\":{\r\n          \"href\":\"https://onedrive.live.com/redir.aspx?cid=c3a40648ad0c9170&page=edit&resid=C3A40648AD0C9170!194479&parId=C3A40648AD0C9170!106\"\r\n        }\r\n      }\r\n    },{\r\n      \"id\":\"0-C3A40648AD0C9170!271532\",\"self\":\"https://www.onenote.com/api/v1.0/me/notes/notebooks/0-C3A40648AD0C9170!271532\",\"createdTime\":\"2017-06-21T19:10:24.127Z\",\"name\":\"ZhengmianHu\",\"createdBy\":\"Ansom Voodoo\",\"lastModifiedBy\":\"Ansom Voodoo\",\"lastModifiedTime\":\"2017-06-26T20:50:20Z\",\"isDefault\":false,\"userRole\":\"Contributor\",\"isShared\":true,\"sectionsUrl\":\"https://www.onenote.com/api/v1.0/me/notes/notebooks/0-C3A40648AD0C9170!271532/sections\",\"sectionGroupsUrl\":\"https://www.onenote.com/api/v1.0/me/notes/notebooks/0-C3A40648AD0C9170!271532/sectionGroups\",\"links\":{\r\n        \"oneNoteClientUrl\":{\r\n          \"href\":\"onenote:https://d.docs.live.net/c3a40648ad0c9170/ansom/Expt.ansom/Personal%20Notebooks/ZhengmianHu\"\r\n        },\"oneNoteWebUrl\":{\r\n          \"href\":\"https://onedrive.live.com/redir.aspx?cid=c3a40648ad0c9170&page=edit&resid=C3A40648AD0C9170!271532&parId=C3A40648AD0C9170!131418\"\r\n        }\r\n      }\r\n    }\r\n  ]\r\n}") -> (0 "error out":errorcluster, 3 "Notebooks LabVIEW":T1)   [LabVIEW 2016]
uses:
  <vilib>/addons/_JKI.lib/Serialization/JSON/JKI JSON Serialization.lvlib
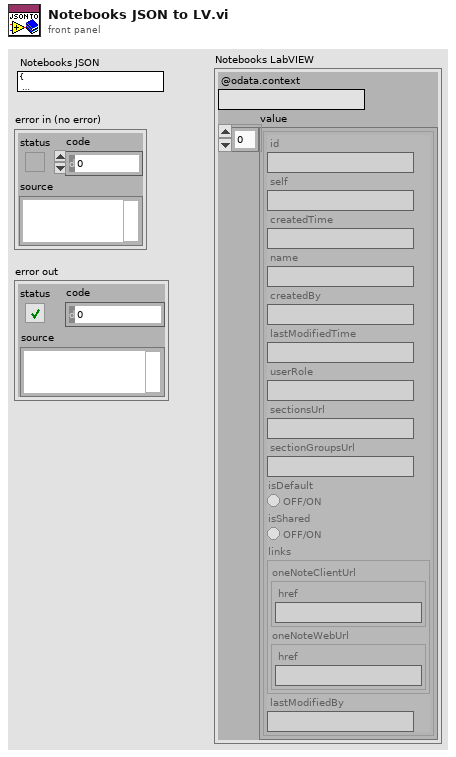
[diagram p1: front panel]
types:
  T1 = cluster{"@odata.context":string, "value":cluster{"id":string, "self":string, "createdTime":string, "name":string, "createdBy":string, "lastModifiedTime":string, "userRole":string, "sectionsUrl":string, "sectionGroupsUrl":string, "isDefault":bool, "isShared":bool, "links":cluster{"oneNoteClientUrl":cluster{"href":string}, "oneNoteWebUrl":cluster{"href":string}}, "lastModifiedBy":string}[]}
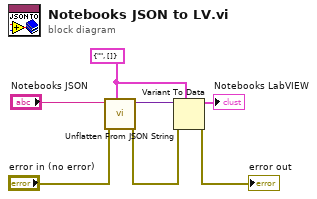
[diagram p0: block diagram]
diagram:
  w5 = T1 {"@odata.context"="", "value"=[]}
  n1 = call <vilib>:"Unflatten From JSON String.vi"("Type and Defaults"=w5, "error in (no error)"="error in (no error)", "JSON String"="Notebooks JSON") -> ("error out"=w3:errorcluster, "Variant"=w6:variant)  [unwired: 7 in]
  n2 = Variant To Data(error in=w3, type=w5, Variant=w6) -> (data=→"Notebooks LabVIEW":T1, error out=→"error out":errorcluster)
